vi "Preference_Panel.vi"(0 "Mode":T3) -> ()   [LabVIEW 2022 SP3]
uses:
  Anemometry Sub Vis/Controls/Server_Comms.ctl
  Anemometry Sub Vis/Controls/Preference_Mode.ctl
  Anemometry Sub Vis/Controls/GMU Gas Line Name.ctl
  Anemometry Sub Vis/File/Setup_Filetype.ctl
  Anemometry Sub Vis/Controls/Overhead.ctl
  ADAM Client/Sub VIs/ADAM Controls/Ch_description_ADAM.ctl
  ADAM Client/Sub VIs/ADAM Controls/Module_type_ADAM.ctl
  ADAM Client/Sub VIs/ADAM Controls/Function_ADAM.ctl
  ADAM Client/Sub VIs/ADAM Controls/Channel_State.ctl
  ADAM Client/Sub VIs/ADAM Controls/Calib_type_ADAM.ctl
  ADAM Client/Sub VIs/ADAM Controls/Address.ctl
  Anemometry Sub Vis/Controls/Serveds.ctl
  <vilib>/Utility/error.llb/Trim Whitespace One-Sided.vi
  Anemometry Sub Vis/Globals/Constants_global.vi
  Anemometry Sub Vis/Globals/Preference_global.vi
  <vilib>/Utility/config.llb/Read Key (Path).vi
  <vilib>/Utility/config.llb/Read Key (String).vi
  <vilib>/Utility/config.llb/Read Key (Boolean).vi
  Anemometry Sub Vis/Globals/Trav_pos_global.vi
  <vilib>/Utility/config.llb/Read Key (U32).vi
  <vilib>/Utility/config.llb/Read Key (Double).vi
  Camera Server/Globals/CamServer global.vi
  <vilib>/Utility/config.llb/Write Key (String).vi
  <vilib>/Utility/config.llb/Write Key (U32).vi
  <vilib>/Utility/config.llb/Write Key (Double).vi
  <vilib>/Utility/config.llb/Write Key (Boolean).vi
  <vilib>/Utility/config.llb/Write Key (I32).vi
  <vilib>/Utility/config.llb/Write Key (Path).vi
  <vilib>/Utility/config.llb/NI_LVConfig.lvlib
panel:
  out "siteString":string
  out "Default Gas Line Name":T1
  in  "Change?":bool
  out "User Name":string
  out "Templates folder":path
  out "Copy of Current User Preferences":path
  in  "Use New Collision Code":bool
  in  "Traverse to Traverse Collision Detection":bool
  in  "IMAQ?":bool
  in  "View Local Cameras Now":bool
  in  "Select Local Cameras to Log":i32[](listbox)
  in  "Log Cameras if available":bool
  in  "MaxDailyEmails":u32=20
  out "auditTrail":string[](array[string])
  out "currentCase":string
  out "prefsPath":path
  in  "DefaultFileExtension":string=".xls"
  in  "Post Processing Machine":bool
  in  "ADAM Setup File":u16(ring) items=["mapTest.xls", "AliGRCvac.xls", "Current_Setup.xls"]
  in  "Rig Setup":u16(ring) items=["All_Rigs", "TestRig", "--New Rig Setup--"]
  in  "Default Traverse Name":u16(ring) items=["None", "--New Traverse Setup--"]
  in  "Data Folder":path
  out "Preferences for computer":string
  in  "Reset Email Counter":bool
  in  "Default Source Establishment Time (s)":dbl=20.0
  in  "% Error From Previous Calib":dbl=0.5 format="%.1f"
  in  "Tunnel Speed Control":bool
  out "This Machine's IP Number":string
  in  "Server port number":u32=3363
  in  "Server address":string
  in  "Server Comms":T2
  in  "OK":bool
  out "Templates":path=path "/G4_2_HD/Applications (Mac OS 9)/EnFlo Software/Anemometry/Anemometry Sub Vis/Templates"
  out "EnFlo SW Preferences":path=path "/G4_2_HD/Applications (Mac OS 9)/LabVIEW 5.1/EnFlo SW Preferences"
  in  "SMTP server IP address":string
  in  "Temperature":string
  in  "Abs Press (mbar)":string
  out "LabVIEW Administrators":string[](array[string])
  in  "FixedUserName":bool caption="Auto?"
  # "Server Computer Peferences"
  # "Email Peferences"
  # "Values come from the Channel named\nLabVIEW:Administrators:\non the ADAM Scan Table. Email addesses are\n in the \"string\" box separated by semi colons."
  # "Camera Peferences"
  # "Multi Run Preferences"
  # "Warning Levels for Autocalibration Changes"
  # "Deg C"
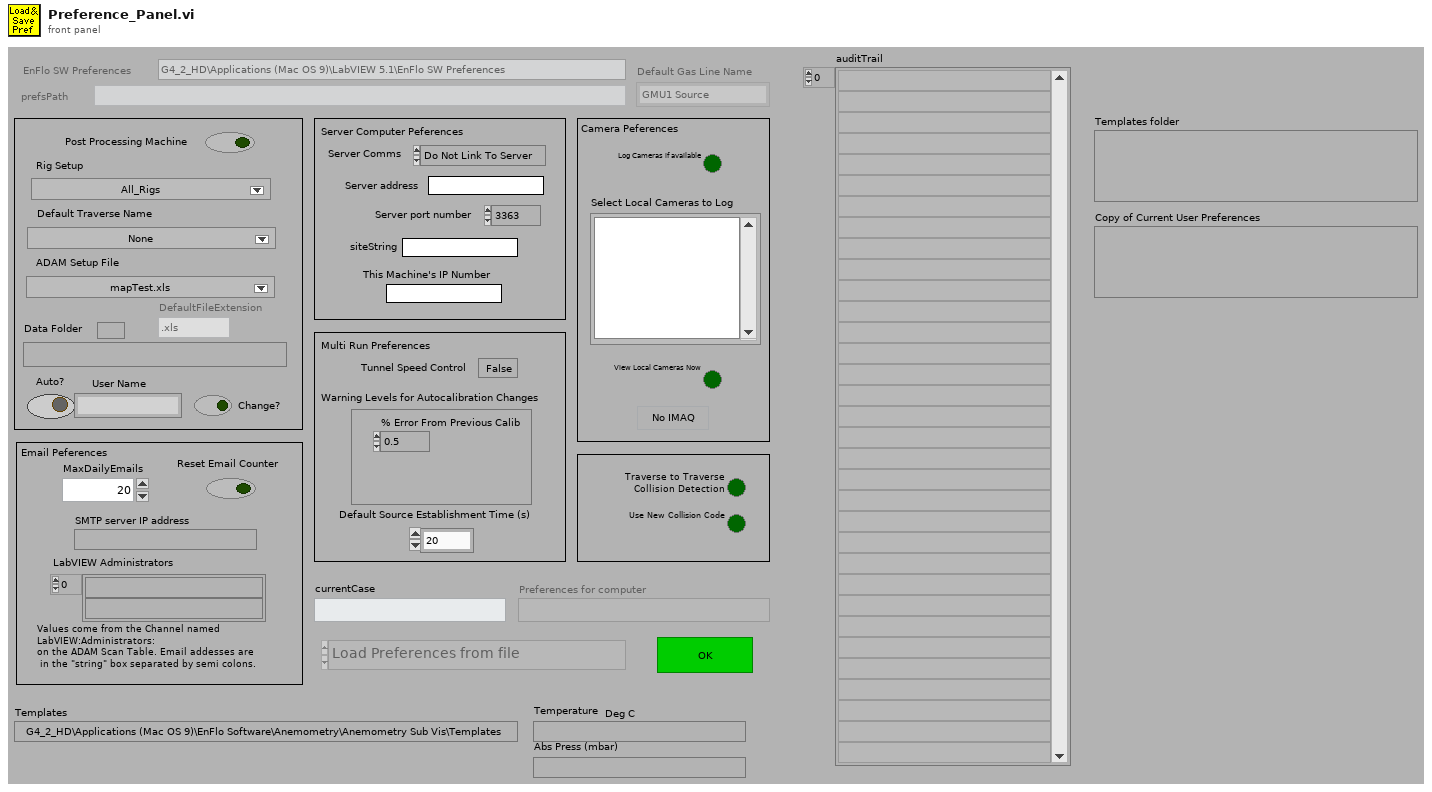
[diagram p1: front panel]
types:
  T1 = typedef "GMU Gas Line Name.ctl" = enum16{"GMU1 Source", "GMU2 Source", "GMU2 Calib", "CPP GRC-A", "CPP GRC-B"}
  T2 = typedef "Server_Comms.ctl" = enum16{"Do Not Link To Server", "Server Link Healthy"}
  T3 = typedef "Preference_Mode.ctl" = enum16{"Load Preferences from file", "Save Preferences to file", "Load, Edit then Save"}
  T4 = enum8{"Enabled", "Disabled", "Disabled and Grayed Out"}
  T5 = typedef "Setup_Filetype.ctl" = enum16{"Measurement Setups", "Calibration Setups", "General", "Results File Plotter Setups", "Speed Calib Tweaks"}
  T6 = enum16{"Zero or one", "One", "Zero or more", "One or more"}
  T7 = typedef "Overhead.ctl" = enum16{"Update total times", "Read Current Overhead", "Re Scale totals to 3 hrs", "Initialise totals to 3hr"}
  T8 = typedef "Calib_type_ADAM.ctl" = string
  T9 = typedef "Module_type_ADAM.ctl" = string
  T10 = typedef "Channel_State.ctl" = enum16{"On", "Off", "Always On", "Always Off"}
  T11 = typedef "Serveds.ctl" = enum16{"Read Global", "Load Global From File"}
  T12 = typedef "NI_LVConfig.lvlib/Config Data RefNum.ctl" = refnum<k1>
  T13 = typedef "LVDateTimeRec.ctl" = cluster{"fractional second":dbl, "second":i32, "minute":i32, "hour":i32, "day of month":i32, "month":i32, "year":i32, "day of week":i32, "day of year":i32, "DST":i32}
  T14 = typedef "camCluster.ctl" = cluster{"cam":string, "URL":string, "ADAMspecs":cluster{"channel":string, "labelText":string, "formatString":string}[]}
  T15 = typedef "Camera enum.ctl" = string
  T16 = cluster{"Label.Text":string, "date/time string":string}[]
  T17 = typedef "Ch_description_ADAM.ctl" = cluster{"Ch Name":string, "Type":T9, "Function":T18, "Ch State":T10, "Calibration type":T8, "A":dbl, "B":dbl, "C":dbl, "D":dbl, "Comments":string, "Address":T19, "String":string, "Duty":u16}
  T18 = typedef "Function_ADAM.ctl" = enum16{"Analogue Input", "Digital Input", "Event counter", "Event rate", "Analogue Output", "Digital Output", "Relay Output"}
  T19 = typedef "Address.ctl" = cluster{"Main":i32, "Ch.":i32, "Sub":i32, "Port Name":string}
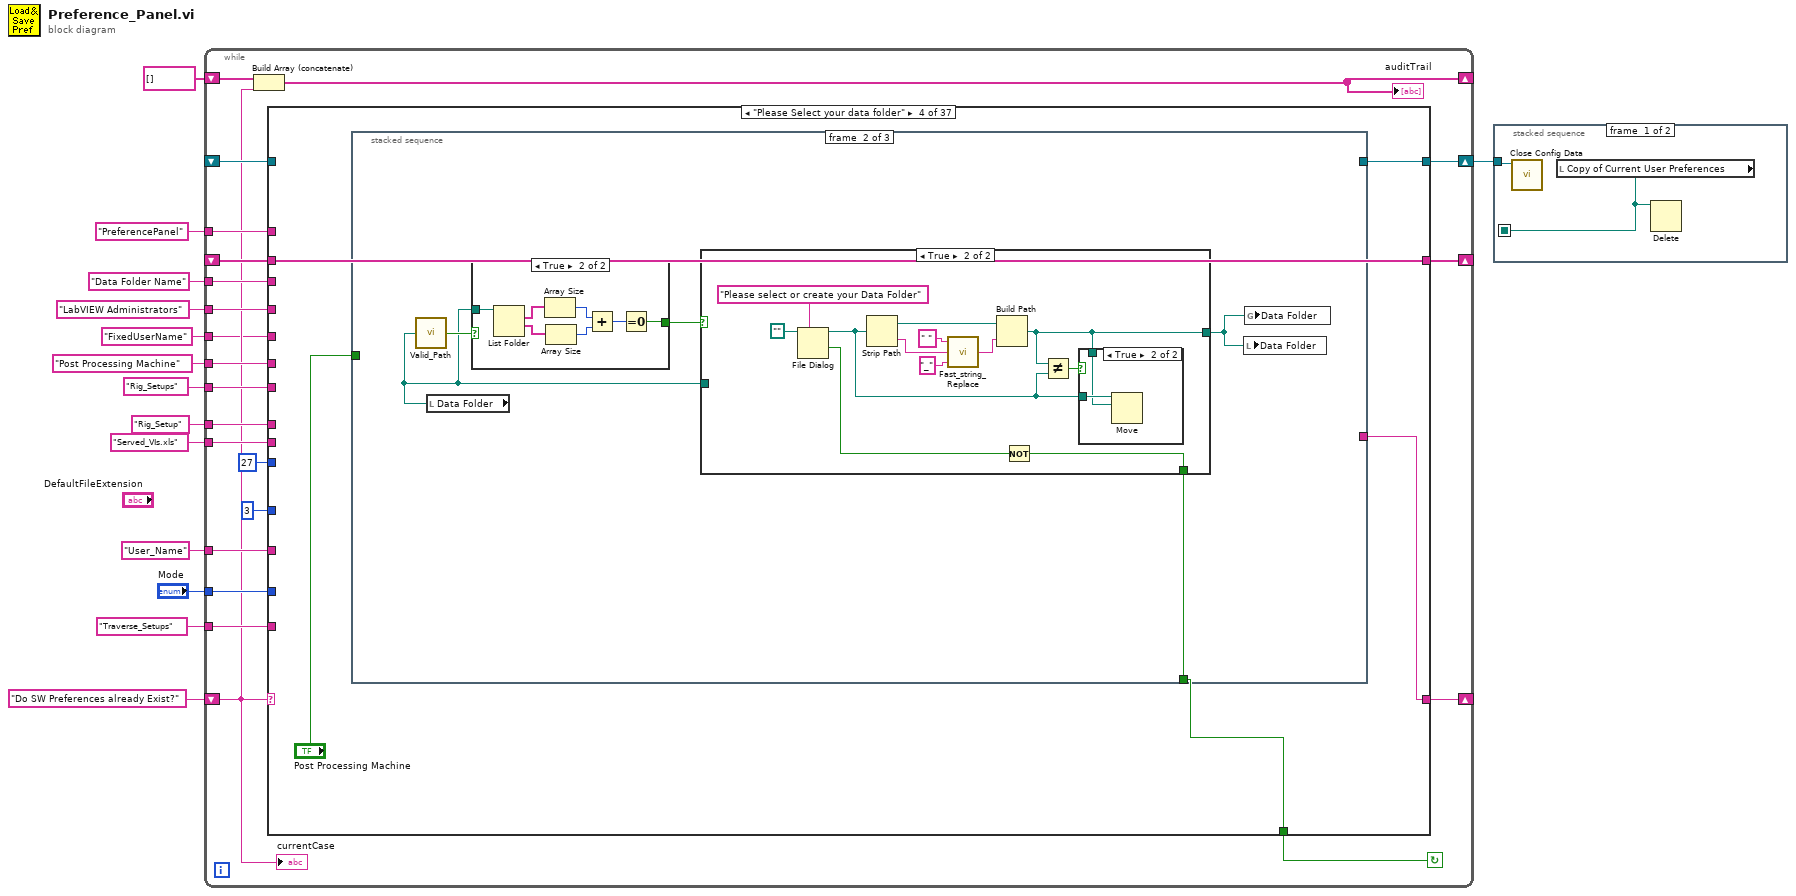
[diagram p0: block diagram]
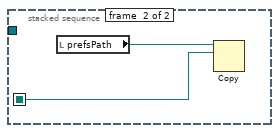
[diagram p2: hidden frame]
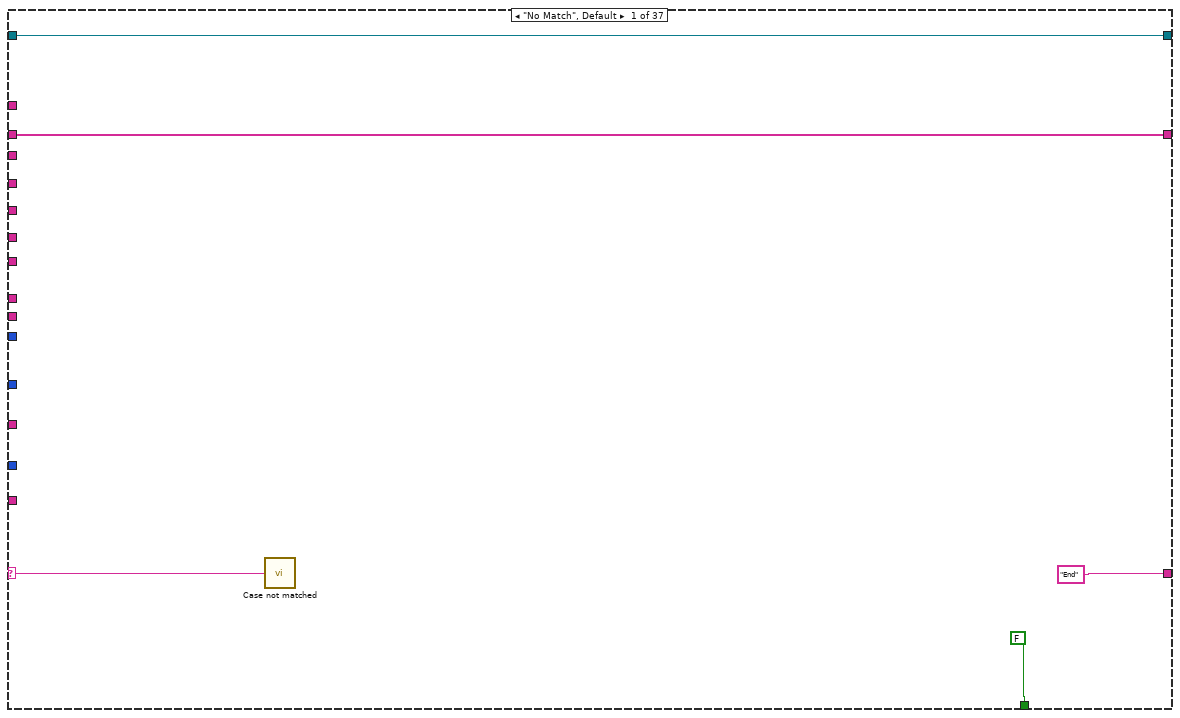
[diagram p3: hidden frame]
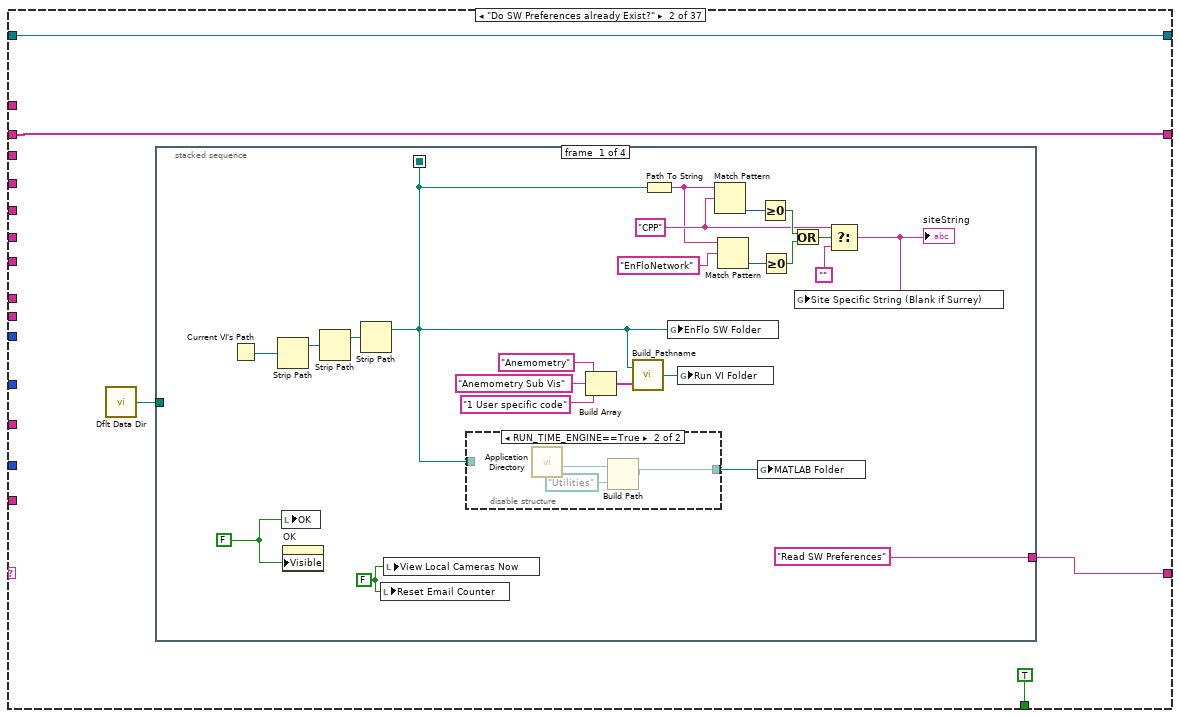
[diagram p4: hidden frame]
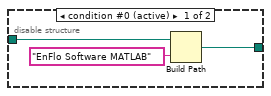
[diagram p5: hidden frame]
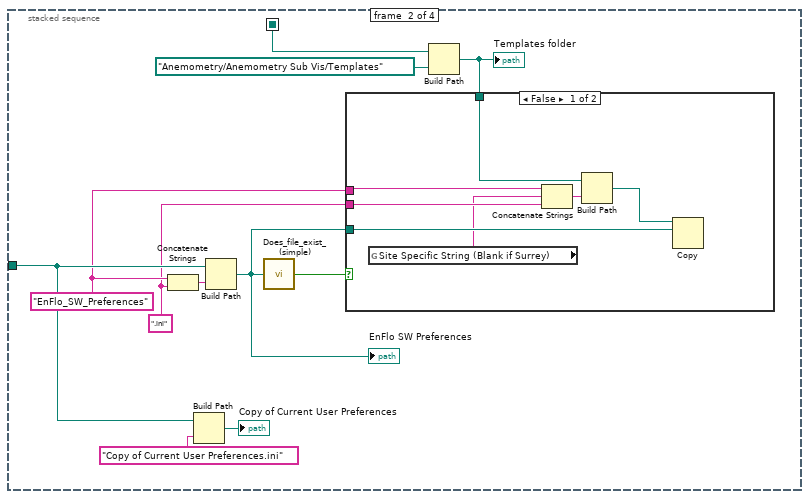
[diagram p6: hidden frame]
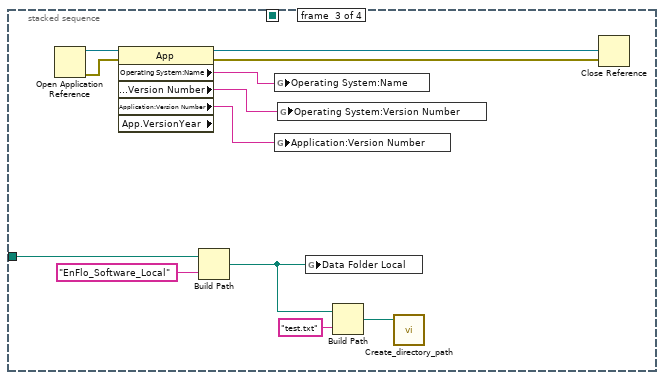
[diagram p8: hidden frame]
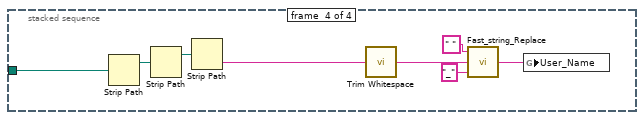
[diagram p9: hidden frame]
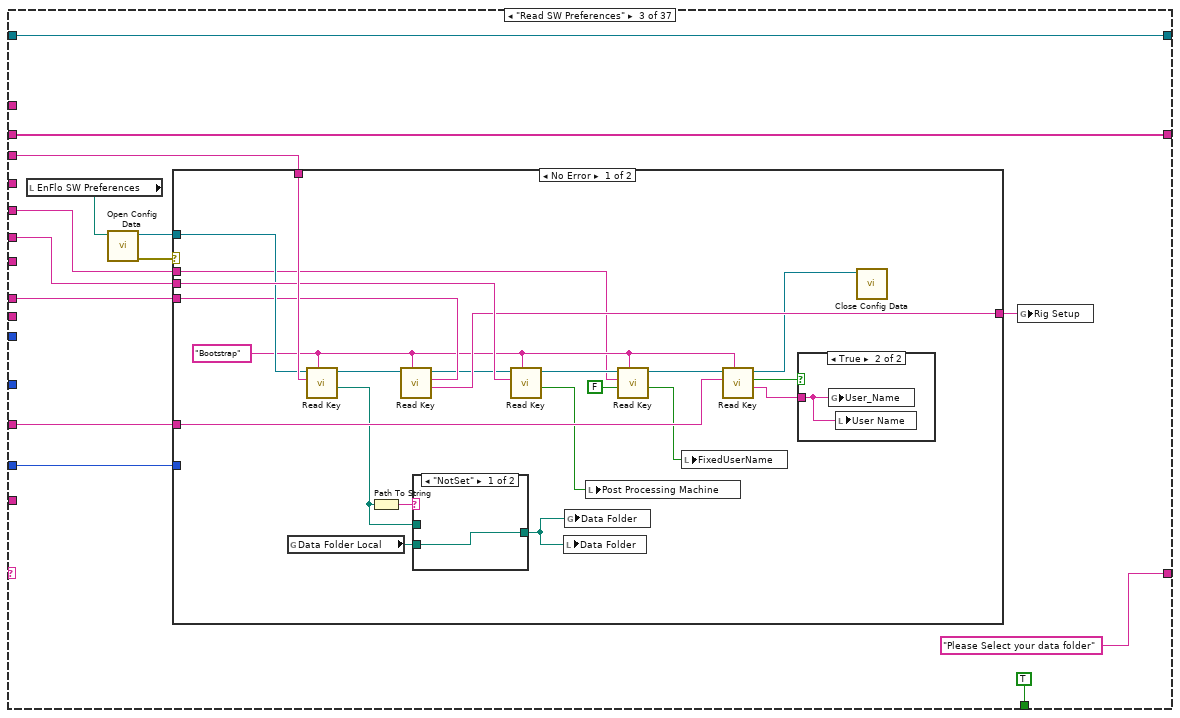
[diagram p10: hidden frame]
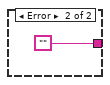
[diagram p13: hidden frame]
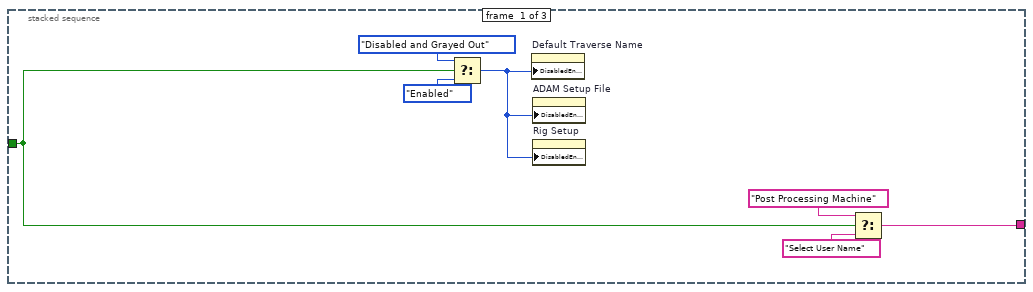
[diagram p14: hidden frame]
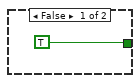
[diagram p15: hidden frame]
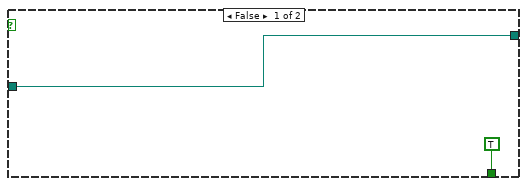
[diagram p16: hidden frame]
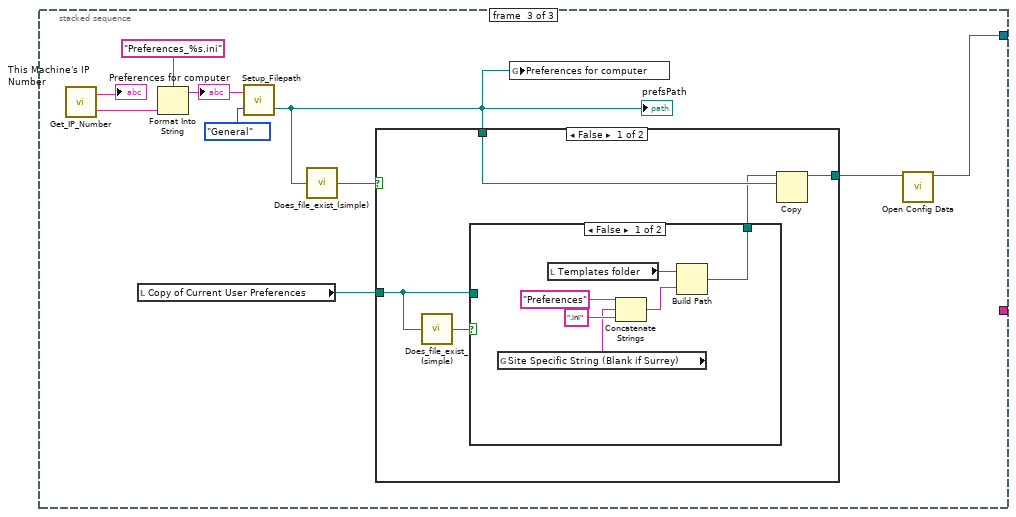
[diagram p18: hidden frame]
diagram:
  n1 = while {
    shift-left: _ -> [w34]
    shift-right: [w35] -> _
    shift-left: "Do SW Preferences already Exist?" -> [w18]
    shift-right: [w19] -> _
    tunnel: "Mode" -> [w33]
    tunnel: "Data Folder Name" ("Label for characters") -> [w32]
    tunnel: "Served_VIs.xls" ("Substring") -> [w31]
    tunnel: "Rig_Setups" ("Folder") -> [w28]
    tunnel: "Traverse_Setups" ("name or relative path") -> [w27]
    tunnel: "Post Processing Machine" ("Label for characters") -> [w26]
    tunnel: "User_Name" ("Label for characters") -> [w25]
    tunnel: "LabVIEW Administrators" -> [w24]
    tunnel: "PreferencePanel" ("section") -> [w23]
    shift-right: [w22] -> w4
    shift-left: _ -> [w21]
    tunnel: "Rig_Setup" ("Label for characters") -> [w20]
    shift-right: [w16] -> _
    shift-left: string[] [] -> [w17]
    tunnel: "FixedUserName" ("key") -> [w15]
    stop <- w36 continue-if-true
    n2 = Build Array (concatenate)(w17, w18) -> (w16:string[])
    "auditTrail" <- w16
    n3 = case shown="\"Please Select your data folder\"" w18 {
      selector: w18 -> [w37 _ _ _ _ _ _ _ _ _ _ _ _ _ _ _ _ _ _ _ _ _ _ _ _ _ _ _ _ _ _ _ _ _ _ _ _]
      tunnel: [FALSE TRUE TRUE w157 TRUE TRUE TRUE TRUE TRUE TRUE TRUE TRUE TRUE TRUE TRUE TRUE TRUE TRUE TRUE TRUE TRUE TRUE TRUE TRUE TRUE TRUE TRUE TRUE TRUE TRUE TRUE TRUE w1012 TRUE TRUE TRUE FALSE] -> w36
      tunnel: ["End" w44 "Please Select your data folder" w154 "Is rig setup blank?" w292 w298 w309 w327 "Update Constants Global" ("f") "Copy Preferences?" "Copy Preferences?" w459 w477 "Install Preference files" "Install Adam table files" "Install Adam setup files" "Choose ADAM Setup file" "Preference files continued" "Variable Names" w653 w689 "Please Enter new  Traverse Setup" w811 "Create Traverse setup" ("f") "Check file permission status" w899 w913 w933 w957 w973 "Save Preference File" "Save SW Preferences" w1134 w1148 "Initialise Globals" "End"] -> w19
      tunnel: [w39 w45 w126 w158 w227 w295 w306 w316 w329 w394 w422 w445 w458 w480 w534 w551 w577 w595 w617 w625 w658 w693 w799 w813 w848 w861 w900 w918 w938 w964 w977 w1000 w1015 w1136 w1149 w1203 w1272] -> w35
      tunnel: w34 -> [w39 w45 w126 w158 w227 w295 w306 w316 w329 w394 w422 w445 w458 w480 w534 w551 w577 w595 w617 w625 _ w693 w799 w813 w848 w861 w900 w918 w938 w964 w977 w1000 w1015 w1136 w1149 w1203 w1272]
      tunnel: w33 -> [_ _ w121 _ w222 _ _ _ _ _ _ _ _ _ _ _ _ _ _ _ w643 _ _ _ _ _ w898 _ _ _ _ _ w1013 _ _ _ _]
      tunnel: w32 -> [_ _ w125 _ w225 _ _ _ _ _ _ _ _ _ _ _ _ _ _ _ _ _ _ _ _ _ _ _ _ _ _ _ _ w1126 _ _ _]
      tunnel: w31 -> [_ _ _ _ _ _ _ _ _ _ _ _ _ _ _ w543 _ _ _ _ _ _ _ _ _ _ _ _ _ _ _ _ _ _ _ w1196 _]
      tunnel: 3 ("lower limit") -> [_ _ _ _ _ _ w303 _ w326 _ _ _ _ _ _ _ _ _ _ _ _ _ _ w810 _ _ _ _ _ _ _ _ _ _ _ _ _]
      tunnel: 27 ("upper limit") -> [_ _ _ _ _ _ w304 _ w325 _ _ _ _ _ _ _ _ _ _ _ _ _ _ w809 _ _ _ _ _ _ _ _ _ _ _ _ _]
      tunnel: w28 -> [_ _ _ _ _ _ _ _ _ w382 w411 _ _ _ _ _ _ _ _ _ _ _ _ _ _ _ _ _ _ _ _ _ _ _ _ _ _]
      tunnel: w27 -> [_ _ _ _ _ _ _ _ _ _ _ _ _ _ _ _ _ _ _ _ _ _ w797 _ w837 _ _ _ _ _ _ _ _ _ _ _ _]
      tunnel: w26 -> [_ _ w124 _ w224 _ _ _ _ _ _ _ _ _ _ _ _ _ _ _ _ _ _ _ _ _ _ _ _ _ _ _ _ w1124 _ _ _]
      tunnel: w25 -> [_ _ w122 _ w223 _ _ _ _ _ _ _ _ _ _ _ _ _ _ _ _ _ _ _ _ _ _ _ _ _ _ _ _ w1122 _ _ _]
      tunnel: w24 -> [_ _ _ _ _ _ _ _ _ _ _ _ _ _ _ _ _ _ _ _ _ _ _ _ _ _ _ _ _ _ _ _ _ _ _ _ _]
      tunnel: w23 -> [_ _ _ _ _ _ _ _ _ _ _ _ _ _ _ _ _ _ _ _ w640 w687 _ _ _ _ _ _ _ _ _ _ w1009 _ _ _ _]
      tunnel: [w38 w42 w120 w156 w221 w294 w297 w308 w321 w380 w402 w427 w450 w475 w524 w540 w562 w587 w603 w619 w638 w686 w788 w805 w834 w856 w896 w910 w930 w953 w972 w998 w1010 w1132 w1147 w1194 w1258] -> w22
      tunnel: w21 -> [w38 w42 w120 _ w221 w294 w297 w308 w321 w380 w402 w427 w450 w475 w524 w540 w562 w587 w603 w619 w638 w686 w788 w805 w834 w856 w896 w910 w930 w953 w972 w998 w1010 w1132 w1147 w1194 w1258]
      tunnel: w20 -> [_ _ w116 _ w220 _ _ _ _ _ _ _ _ _ _ _ _ _ _ _ _ _ _ _ _ _ _ _ _ _ _ _ _ w1116 _ _ _]
      tunnel: w15 -> [_ _ w114 _ _ _ _ _ _ _ _ _ _ _ _ _ _ _ _ _ _ _ _ _ _ _ _ _ _ _ _ _ _ w1112 _ _ _]
      frame "No Match", Default {
        n4 = call "Case not matched.vi"("Case Name not Matched"=w37) -> ()
      }
      frame "Do SW Preferences already Exist?" {
        n5 = call <vilib>:"Dflt Data Dir.vi"() -> ("App:Default Data Directory"=w43:path)
        n6 = stacked-sequence {
          seq-local: [w49 _ _ _] -> [_ w81 _ _]
          tunnel: ["Read SW Preferences" _ _ _] -> w44
          tunnel: w43 -> [_ w84 w97 w107]
          frame #0 {
            w51 = "CPP" ("regular expression")
            w62 = FALSE ("Reset Email Counter")
            w69 = FALSE ("OK")
            n7 = Current VI's Path() -> (path=w60:path)
            n8 = Strip Path(path=w60) -> (stripped path=w59:path)  [unwired: 1 out]
            n9 = local write "OK"(w69) -> ()
            n10 = property on="OK" class="Bool (strict)"("Visible"=w69) -> ()  [unwired: 2 in, 2 out]
            n11 = Strip Path(path=w59) -> (stripped path=w58:path)  [unwired: 1 out]
            n12 = Strip Path(path=w58) -> (stripped path=w49:path)  [unwired: 1 out]
            n13 = local write "Reset Email Counter"(w62) -> ()
            n14 = local write "View Local Cameras Now"(w62) -> ()
            n15 = disable-structure shown="RUN_TIME_ENGINE==True" {
              disable-tunnel: [w71 w75] -> w63
              disable-tunnel: w49 -> [w70 _]
              frame condition #0 (active) {
                n16 = Build Path(base path=w70, name or relative path="EnFlo Software MATLAB") -> (appended path=w71:path)
              }
              frame condition #1 {
                n17 = call <vilib>:"Application Directory.vi"() -> ("Application Directory"=w74:path)
                n18 = Build Path(base path=w74, name or relative path=path "Utilities") -> (appended path=w75:path)
              }
            }
            n19 = Build Array("Anemometry" ("name or relative path"), "Anemometry Sub Vis" ("name or relative path"), "1 User specific code" ("name or relative path")) -> (w64:string[])
            n20 = call "Build_Pathname.vi"("PathElements"=w64, "PathnameIn"=w49) -> ("AppendedPath"=w68:path)
            n21 = Path To String(path=w49) -> (string=w48:string)
            n22 = global write "Constants_global.vi" "EnFlo SW Folder"(w49) -> ()
            n23 = global write "Constants_global.vi" "Run VI Folder"(w68) -> ()
            n24 = Match Pattern(string=w48, regular expression=w51) -> (offset past match=w57:i32)  [unwired: 1 in, 3 out]
            n25 = Match Pattern(string=w48, regular expression="EnFloNetwork") -> (offset past match=w56:i32)  [unwired: 1 in, 3 out]
            n26 = global write "Constants_global.vi" "MATLAB Folder"(w63) -> ()
            n27 = Greater Or Equal To 0?(x=w57) -> (x >= 0?=w55:bool)
            n28 = Greater Or Equal To 0?(x=w56) -> (x >= 0?=w54:bool)
            n29 = Or(x=w55, y=w54) -> (x .or. y?=w53:bool)
            n30 = Select(t=w51, s=w53, f="") -> (s? t:f=w47:string)
            "siteString" <- w47
            n31 = global write "Preference_global.vi" "Site Specific String (Blank if Surrey)"(w47) -> ()
          }
          frame #1 {
            w76 = ".ini" ("name or relative path")
            w78 = "EnFlo_SW_Preferences" ("name or relative path")
            n32 = Concatenate Strings(w78, w76) -> (w77:string)
            n33 = Build Path(base path=w84, name or relative path="Copy of Current User Preferences.ini") -> (appended path=→"Copy of Current User Preferences":path)
            n34 = Build Path(base path=w84, name or relative path=w77) -> (appended path=w82:path)
            "EnFlo SW Preferences" <- w82
            n35 = call "Does_file_exist_(simple).vi"("Pathname"=w82) -> ("exists?"=w83:bool)
            n36 = Build Path(base path=w81, name or relative path=path "Anemometry/Anemometry Sub Vis/Templates" ("appended path")) -> (appended path=w79:path)
            "Templates folder" <- w79
            n37 = case shown="False" w83 {
              tunnel: w82 -> [w92 _]
              tunnel: w79 -> [w91 _]
              tunnel: w78 -> [w89 _]
              tunnel: w76 -> [w88 _]
              frame False {
                n38 = global read "Preference_global.vi" "Site Specific String (Blank if Surrey)"() -> (w87:string)
                n39 = Concatenate Strings(w89, w87, w88) -> (w90:string)
                n40 = Build Path(base path=w91, name or relative path=w90) -> (appended path=w93:path)
                n41 = Copy(10:w92, 11:w93) -> ()  [unwired: 3 in, 3 out]
              }
              frame True {
              }
            }
          }
          frame #2 {
            n42 = Open Application Reference() -> (0:w102:errorcluster, 3:w105:refnum<vi>)  [unwired: 1 in, 3 out]
            n43 = property class="App" props=["Operating System:Name", "Operating System:Version Number", "Application:Version Number", "App.VersionYear"](reference=w105, error in=w102) -> (reference out=w104:refnum<vi>, error out=w103:errorcluster, "Operating System:Name"=w99:string, "Operating System:Version Number"=w101:string, "Application:Version Number"=w100:string)  [unwired: 1 out]
            n44 = Build Path(base path=w97, name or relative path="EnFlo_Software_Local" ("element")) -> (appended path=w96:path)
            n45 = global write "Preference_global.vi" "Operating System:Name"(w99) -> ()
            n46 = global write "Preference_global.vi" "Application:Version Number"(w100) -> ()
            n47 = global write "Preference_global.vi" "Operating System:Version Number"(w101) -> ()
            n48 = global write "Constants_global.vi" "Data Folder Local"(w96) -> ()
            n49 = Build Path(base path=w96, name or relative path="test.txt") -> (appended path=w94:path)
            n50 = call "Create_directory_path.vi"("Path name"=w94) -> ()  [unwired: 2 in, 2 out]
            n51 = Close Reference(reference=w104, error in (no error)=w103) -> ()  [unwired: 1 out]
          }
          frame #3 {
            n52 = Strip Path(path=w107) -> (stripped path=w109:path)  [unwired: 1 out]
            n53 = Strip Path(path=w109) -> (stripped path=w108:path)  [unwired: 1 out]
            n54 = Strip Path(path=w108) -> (name=w106:string)  [unwired: 1 out]
            n55 = call <vilib>:"Trim Whitespace.vi"("string"=w106) -> ("trimmed string"=w110:string)  [unwired: 1 in]
            n56 = call "Fast_string_Replace.vi"("Replace match with:"="_", "Input String"=w110, "matchThis"=" " ("regular expression")) -> ("Output String"=w111:string)  [unwired: 1 in, 1 out]
            n57 = global write "Preference_global.vi" "User_Name"(w111) -> ()
          }
        }
      }
      frame "Read SW Preferences" {
        n58 = local read "EnFlo SW Preferences"() -> (w117:path)
        n59 = call <vilib>:"Open Config Data.vi"("configuration file path"=w117) -> ("error out"=w118:errorcluster, "refnum"=w119:T12)  [unwired: 8 in, 1 out]
        n60 = case shown="No Error" w118 {
          tunnel: w125 -> [w149 _]
          tunnel: w124 -> [w148 _]
          tunnel: [w147 ""] -> w123
          tunnel: w122 -> [w146 _]
          tunnel: w121 -> [_ _]
          tunnel: w119 -> [w145 _]
          tunnel: w116 -> [w144 _]
          tunnel: w114 -> [w129 _]
          frame No Error {
            w130 = "Bootstrap"
            n61 = global read "Constants_global.vi" "Data Folder Local"() -> (w136:path)
            n62 = call-poly <vilib>:"Read Key.vi"("section"=w130, "key"=w149, "refnum"=w145) -> ("value"=w134:path, "refnum out"=w140:T12)  [unwired: 5 in, 2 out]
            n63 = Path To String(path=w134) -> (string=w137:string)
            n64 = call-poly <vilib>:"Read Key.vi"("section"=w130, "key"=w144, "refnum"=w140) -> ("value"=w147:string, "refnum out"=w139:T12)  [unwired: 5 in, 2 out]
            n65 = case shown="\"NotSet\"" w137 {
              tunnel: w136 -> [w150 _]
              tunnel: [w150 w151] -> w135
              tunnel: w134 -> [_ w151]
              frame "NotSet" {
              }
              frame "Set", Default {
              }
            }
            n66 = call-poly <vilib>:"Read Key.vi"("section"=w130, "key"=w148, "refnum"=w139) -> ("value"=w143:bool, "refnum out"=w133:T12)  [unwired: 5 in, 2 out]
            n67 = local write "Data Folder"(w135) -> ()
            n68 = global write "Constants_global.vi" "Data Folder"(w135) -> ()
            n69 = local write "Post Processing Machine"(w143) -> ()
            n70 = call-poly <vilib>:"Read Key.vi"("section"=w130, "default value"=FALSE, "key"=w129, "refnum"=w133) -> ("value"=w128:bool, "refnum out"=w132:T12)  [unwired: 4 in, 2 out]
            n71 = local write "FixedUserName"(w128) -> ()
            n72 = call-poly <vilib>:"Read Key.vi"("section"=w130, "key"=w146, "refnum"=w132) -> ("value"=w141:string, "found?"=w142:bool, "refnum out"=w138:T12)  [unwired: 5 in, 1 out]
            n73 = case shown="True" w142 {
              tunnel: w141 -> [_ w152]
              frame False {
              }
              frame True {
                n74 = global write "Preference_global.vi" "User_Name"(w152) -> ()
                n75 = local write "User Name"(w152) -> ()
              }
            }
            n76 = call <vilib>:"Close Config Data.vi"("refnum"=w138) -> ()  [unwired: 9 in, 2 out]
          }
          frame Error {
          }
        }
        n77 = global write "Preference_global.vi" "Rig Setup"(w123) -> ()
      }
      frame "Please Select your data folder" {
        n78 = stacked-sequence {
          tunnel: [_ w170 _] -> w157
          tunnel: "Post Processing Machine" -> [w159 _ _]
          tunnel: [_ _ w199] -> w156
          tunnel: [w160 _ _] -> w154
          frame #0 {
            n79 = Select(t=T4."Disabled and Grayed Out" ("Disabled"), s=w159, f=T4."Enabled" ("Disabled")) -> (s? t:f=w165:T4)
            n80 = property on="Default Traverse Name" class="Ring (strict)"("DisabledEnum"=w165) -> ()  [unwired: 2 in, 2 out]
            n81 = property on="ADAM Setup File" class="Ring (strict)"("DisabledEnum"=w165) -> ()  [unwired: 2 in, 2 out]
            n82 = property on="Rig Setup" class="Ring (strict)"("DisabledEnum"=w165) -> ()  [unwired: 2 in, 2 out]
            n83 = Select(t="Post Processing Machine", s=w159, f="Select User Name") -> (s? t:f=w160:string)
          }
          frame #1 {
            n84 = local read "Data Folder"() -> (w166:path)
            n85 = call "Valid_Path.vi"("Filename"=w166) -> ("Valid Path?"=w168:bool)
            n86 = case shown="True" w168 {
              tunnel: [TRUE ("status") w172] -> w167
              tunnel: w166 -> [_ w178]
              frame False {
              }
              frame True {
                n87 = List Folder(path=w178) -> (filenames=w176:string[], folder names=w177:string[])  [unwired: 1 in, 4 out]
                n88 = Array Size(array=w176) -> (size(s)=w174:i32)
                n89 = Array Size(array=w177) -> (size(s)=w175:i32)
                n90 = Add(x=w174, y=w175) -> (x+y=w173:i32)
                n91 = Equal To 0?(x=w173) -> (x = 0?=w172:bool)
              }
            }
            n92 = case shown="True" w167 {
              tunnel: [w180 w183] -> w169
              tunnel: w166 -> [w180 _]
              tunnel: [TRUE w181] -> w170
              frame False {
              }
              frame True {
                n93 = File Dialog(7:"Please select or create your Data Folder" ("prompt"), 11:path "") -> (1:w182:bool, 3:w184:path)  [unwired: 1 in, 6 out]
                n94 = Strip Path(path=w184) -> (stripped path=w188:path, name=w187:string)
                n95 = call "Fast_string_Replace.vi"("Replace match with:"="_", "Input String"=w187, "matchThis"=" " ("regular expression")) -> ("Output String"=w186:string)  [unwired: 1 in, 1 out]
                n96 = Build Path(base path=w188, name or relative path=w186) -> (appended path=w183:path)
                n97 = Not(x=w182) -> (.not. x?=w181:bool)
                n98 = Not Equal?(x=w183, y=w184) -> (x != y?=w185:bool)
                n99 = case shown="True" w185 {
                  tunnel: w184 -> [_ w194]
                  tunnel: w183 -> [_ w193]
                  frame False {
                  }
                  frame True {
                    n100 = Move(source path=w194, 10:w193) -> ()  [unwired: 1 in, 5 out]
                  }
                }
              }
            }
            n101 = local write "Data Folder"(w169) -> ()
            n102 = global write "Constants_global.vi" "Data Folder"(w169) -> ()
          }
          frame #2 {
            n103 = call "Get_IP_Number.vi"() -> ("bestAvailableName"=w203:string, "IP Number"=→"This Machine's IP Number":string)
            n104 = local read "Copy of Current User Preferences"() -> (w196:path)
            n105 = Format Into String(format string="Preferences_%s.ini" ("name or relative path"), w203) -> (resulting string=w204:string)  [unwired: 2 in, 1 out]
            "Preferences for computer" <- w204
            n106 = call "Setup_Filepath.vi"("Setup File Type"=Setup_Filetype."General", "Filename in"=w204) -> ("Filename Out"=w195:path)  [unwired: 1 out]
            "prefsPath" <- w195
            n107 = call "Does_file_exist_(simple).vi"("Pathname"=w195) -> ("exists?"=w198:bool)
            n108 = case shown="False" w198 {
              tunnel: w195 -> [w208 w217]
              tunnel: [w209 w217] -> w197
              tunnel: w196 -> [w205 _]
              frame False {
                n109 = call "Does_file_exist_(simple).vi"("Pathname"=w205) -> ("exists?"=w207:bool)
                n110 = case shown="False" w207 {
                  tunnel: [w214 w216] -> w206
                  tunnel: w205 -> [_ w216]
                  frame False {
                    n111 = global read "Preference_global.vi" "Site Specific String (Blank if Surrey)"() -> (w210:string)
                    n112 = local read "Templates folder"() -> (w215:path)
                    n113 = Concatenate Strings("Preferences", w210, ".ini") -> (w211:string)
                    n114 = Build Path(base path=w215, name or relative path=w211) -> (appended path=w214:path)
                  }
                  frame True {
                  }
                }
                n115 = Copy(10:w208, 11:w206) -> (3:w209:path)  [unwired: 3 in, 2 out]
              }
              frame True {
              }
            }
            n116 = global write "Preference_global.vi" "Preferences for computer"(w195) -> ()
            n117 = call <vilib>:"Open Config Data.vi"("configuration file path"=w197) -> ("refnum"=w199:T12)  [unwired: 8 in, 2 out]
          }
        }
      }
      frame "Select User Name" {
        n118 = local read "Post Processing Machine"() -> (w218:bool)
        n119 = stacked-sequence {
          seq-local: [w231 _ _ _] -> [_ _ w268 _]
          seq-local: [_ w247 _ _] -> [_ _ w258 _]
          tunnel: w225 -> [_ _ _ _]
          tunnel: w224 -> [_ _ _ _]
          tunnel: w223 -> [_ _ _ _]
          tunnel: "Add New User Name" -> [w230 _ w272 _]
          tunnel: w222 -> [_ w248 _ _]
          tunnel: w220 -> [_ _ _ _]
          tunnel: w218 -> [_ w246 _ _]
          frame #0 {
            n120 = Get Date/Time In Seconds() -> (seconds since 1Jan1904=w245:timestamp)
            n121 = global read "Constants_global.vi" "Data Folder"() -> (w238:path)
            n122 = Seconds To Date/Time(time stamp (now)=w245) -> (date time rec=w244:T13)  [unwired: 1 in]
            n123 = Unbundle By Name(w244) -> ("year"=w243:i32)
            n124 = Decrement(x=w243) -> (x-1=w242:i32)
            n125 = Number To Decimal String(number=w242) -> (decimal integer string=w237:string)  [unwired: 1 in]
            n126 = Number To Decimal String(number=w243) -> (decimal integer string=w241:string)  [unwired: 1 in]
            n127 = global read "Preference_global.vi" "Rig Setup"() -> (w229:string)
            n128 = Build Path(base path=w238, name or relative path=w241) -> (appended path=w240:path)
            n129 = Build Path(base path=w238, name or relative path=w237) -> (appended path=w236:path)
            n130 = Build Path(base path=w240, name or relative path=w229) -> (appended path=w239:path)
            n131 = Build Path(base path=w236, name or relative path=w229) -> (appended path=w235:path)
            n132 = List Folder(path=w239) -> (folder names=w234:string[])  [unwired: 3 in, 3 out]
            n133 = List Folder(path=w235) -> (folder names=w233:string[])  [unwired: 3 in, 3 out]
            n134 = Build Array (concatenate)(w234, w233, w230) -> (w232:string[])
            n135 = call "Analyse_string_array.vi"("String array"=w232) -> ("Unique strings"=w231:string[])  [unwired: 1 in, 1 out]
          }
          frame #1 {
            n136 = case shown="False" w246 {
              tunnel: w248 -> [w255 _]
              tunnel: [w251 FALSE] -> w247
              frame False {
                n137 = Equal?(x=Preference_Mode."Load Preferences from file" ("Mode"), y=w255) -> (x = y?=w253:bool)
                n138 = local read "FixedUserName"() -> (w249:bool)
                n139 = Compound Arithmetic op=AND(w253, invert w249) -> (w250:bool)
                n140 = local read "Change?"() -> (w252:bool)
                n141 = Or(x=w250, y=w252) -> (x .or. y?=w251:bool)
              }
              frame True {
              }
            }
          }
          frame #2 {
            n142 = global read "Preference_global.vi" "User_Name"() -> (w269:string)
            n143 = call "Get_IP_Number.vi"() -> ("bestAvailableName"=w261:string, "IP Number"=w262:string)
            n144 = local write "This Machine's IP Number"(w262) -> ()
            n145 = Search 1D Array(1D array=w268, element=w269) -> (index of element=w267:i32)  [unwired: 1 in]
            n146 = Format Into String(format string="Preferences_%s.ini" ("name or relative path"), w261) -> (resulting string=w260:string)  [unwired: 2 in, 1 out]
            n147 = local write "Preferences for computer"(w260) -> ()
            n148 = Less Than 0?(x=w267) -> (x < 0?=w266:bool)
            n149 = Select(t=nan ("Timeout (s)"), s=w266, f=60.0 ("Timeout (s)")) -> (s? t:f=w263:dbl)
            n150 = case shown="True" w258 {
              tunnel: [w273 w280] -> w270
              tunnel: w269 -> [w273 w279]
              tunnel: w268 -> [_ w278]
              tunnel: w263 -> [_ w277]
              frame False {
              }
              frame True {
                n151 = Build Array(w279) -> (w283:string[])
                n152 = call "Select_Strings.vi"("Timeout (s)"=w277, "Available Ch names"=w278, "Message"="Please Select User Name", "Selector mode"=T6."One", "Desired Ch names (in)"=w283) -> ("Cancel"=w275:bool, "Selected Channel Names"=w281:string[], "Timed out?"=w276:bool)  [unwired: 1 out]
                n153 = Compound Arithmetic op=AND(invert w276, w275) -> (w274:bool)
                n154 = Index Array(array=w281) -> (element=w280:string)  [unwired: 1 in]
                n155 = Stop(stop? (T)=w274) -> ()
              }
            }
            n156 = Equal?(x=w270, y=w272) -> (x = y?=w271:bool)
            n157 = case shown="False" w271 {
              tunnel: [w285 w286] -> w257
              tunnel: w270 -> [w285 _]
              frame False {
              }
              frame True {
                n158 = call "Input_String_Dialog.vi"("Message to user"="Please Enter User Name") -> ("Output string"=w286:string)  [unwired: 1 in, 1 out]
              }
            }
            "User Name" <- w257
            n159 = global write "Preference_global.vi" "User_Name"(w257) -> ()
          }
          frame #3 {
            n160 = local write "Change?"(FALSE ("Change?")) -> ()
          }
        }
      }
      frame "Is rig setup blank?" {
        n161 = global read "Preference_global.vi" "Rig Setup"() -> (w289:string)
        n162 = Empty String/Path?(string/path=w289) -> (empty?=w290:bool)
        n163 = Select(t="Update Rig setup menu ring", s=w290, f="Check Rig Setup name" ("t")) -> (s? t:f=w292:string)
      }
      frame "Check Rig Setup name" {
        n164 = global read "Preference_global.vi" "Rig Setup"() -> (w299:string)
        n165 = String Length(string=w299) -> (length=w305:i32)
        n166 = In Range and Coerce(upper limit=w304, x=w305, lower limit=w303) -> (In Range?=w302:bool)  [unwired: 1 out]
        n167 = Select(t="Please Enter New Rig Name", s=w302, f="Question Data Folder") -> (s? t:f=w298:string)
      }
      frame "Question Data Folder" {
        n168 = local read "Data Folder"() -> (w315:path)
        n169 = Format Into String(format string="Is the Data Folder\n%s\nCorrect?" ("message"), w315) -> (resulting string=w313:string)  [unwired: 2 in, 1 out]
        n170 = Two Button Dialog(message=w313, 1:"No, let me change it" ("F button name (\"Cancel\")"), 2:"Yes" ("T button name (\"OK\")")) -> (T button?=w310:bool)
        n171 = case shown="True" w310 {
          tunnel: ["Please Select your data folder" "Please Enter New Rig Name"] -> w309
          frame False {
            n172 = local write "Data Folder"(path "") -> ()
          }
          frame True {
          }
        }
      }
      frame "Please Enter New Rig Name" {
        n173 = global read "Preference_global.vi" "Rig Setup"() -> (w323:string)
        n174 = String Length(string=w323) -> (length=w328:i32)
        n175 = In Range and Coerce(upper limit=w325, x=w328, lower limit=w326) -> (In Range?=w324:bool)  [unwired: 1 out]
        n176 = case shown="True" w324 {
          tunnel: w323 -> [w335 w378]
          tunnel: [w331 "Update Rig setup menu ring"] -> w327
          tunnel: [w332 w378] -> w322
          tunnel: w326 -> [w334 _]
          tunnel: w325 -> [w333 _]
          frame False {
            n177 = stacked-sequence {
              seq-local: [w336 _] -> [_ w361]
              seq-local: [w343 _] -> [_ _]
              tunnel: w335 -> [w345 _]
              tunnel: w334 -> [w356 _]
              tunnel: w333 -> [w342 w359]
              tunnel: [_ w364] -> w332
              tunnel: [w348 _] -> w331
              frame #0 {
                n178 = Match Pattern(string=w345, regular expression="-") -> (before substring=w344:string, after substring=w343:string)  [unwired: 3 out]
                n179 = String Length(string=w343) -> (length=w341:i32)
                n180 = Subtract(x=w342, y=w341) -> (x-y=w340:i32)
                n181 = Format Into String(format string="Please Enter a Rig Name.\n It must be between %d and %d Characters" ("Message to user"), w356, w340) -> (resulting string=w355:string)  [unwired: 2 in, 1 out]
                n182 = call "Input_String_Dialog.vi"("Value"=w344, "Message to user"=w355) -> ("Ok Out"=w351:bool, "Output string"=w352:string)
                n183 = call "Fast_string_Replace.vi"("Replace match with:"="_", "Input String"=w352, "matchThis"=" " ("regular expression")) -> ("Output String"=w337:string)  [unwired: 1 in, 1 out]
                n184 = Select(t="Please Enter New Rig Name", s=w351, f="Save Preference File") -> (s? t:f=w348:string)
                n185 = call "Fast_string_Replace.vi"("Replace match with:"="_", "Input String"=w337, "matchThis"="-" ("regular expression")) -> ("Output String"=w336:string)  [unwired: 1 in, 1 out]
              }
              frame #1 {
                n186 = String Length(string=w361) -> (length=w360:i32)
                n187 = Subtract(x=w359, y=w360) -> (x-y=w358:i32)
                n188 = Format Into String(format string="Please Enter a Rig Machine identifier if more than one machine per Rig.\n(Leave Blank for Rigs only using one Machine.)\nMust be less than %d Characters." ("Message to user"), w358) -> (resulting string=w357:string)  [unwired: 2 in, 1 out]
                n189 = call "Input_String_Dialog.vi"("Value"="", "Message to user"=w357) -> ("Output string"=w370:string)  [unwired: 1 out]
                n190 = call "Fast_string_Replace.vi"("Replace match with:"="_", "Input String"=w370, "matchThis"=" " ("regular expression")) -> ("Output String"=w366:string)  [unwired: 1 in, 1 out]
                n191 = call "Fast_string_Replace.vi"("Replace match with:"="_", "Input String"=w366, "matchThis"="-" ("regular expression")) -> ("Output String"=w363:string)  [unwired: 1 in, 1 out]
                n192 = Empty String/Path?(string/path=w363) -> (empty?=w365:bool)
                n193 = case shown="False" w365 {
                  tunnel: [w373 w377] -> w364
                  tunnel: w361 -> [w376 w377]
                  tunnel: w363 -> [w374 _]
                  frame False {
                    n194 = Concatenate Strings(w376, "-" ("string"), w374) -> (w373:string)
                  }
                  frame True {
                  }
                }
              }
            }
          }
          frame True {
          }
        }
        n195 = global write "Preference_global.vi" "Rig Setup"(w322) -> ()
      }
      frame "Update Rig setup menu ring" {
        n196 = local read "Data Folder"() -> (w385:path)
        n197 = Build Path(base path=w385, name or relative path="Preferences") -> (appended path=w384:path)
        n198 = Build Path(base path=w384, name or relative path=w382) -> (appended path=w383:path)
        n199 = List Folder(path=w383) -> (folder names=w381:string[])  [unwired: 1 in, 5 out]
        n200 = Build Array (concatenate)(w381, "--New Rig Setup--") -> (w387:string[])
        n201 = global read "Preference_global.vi" "Rig Setup"() -> (w391:string)
        n202 = Search 1D Array(1D array=w387, element=w391) -> (index of element=w390:i32)  [unwired: 1 out]
        n203 = case shown="-1" w390 {
          selector: w390 -> [w396 _]
          tunnel: [w396 0] -> w393
          tunnel: w387 -> [w397 w400]
          tunnel: w391 -> [_ w399]
          tunnel: [w397 w398] -> w389
          frame 0, Default {
          }
          frame -1 {
            n204 = Build Array (concatenate)(w399, w400) -> (w398:string[])
          }
        }
        n205 = local write "Rig Setup"(w393) -> ()
        n206 = property on="Rig Setup" class="Ring (strict)"("Strings []"=w389) -> ()  [unwired: 2 in, 2 out]
      }
      frame "Update Constants Global" {
        n207 = global read "Constants_global.vi" "Data Folder"() -> (w409:path)
        n208 = Build Path(base path=w409, name or relative path="Preferences") -> (appended path=w412:path)
        n209 = global read "Preference_global.vi" "Rig Setup"() -> (w410:string)
        n210 = Build Path(base path=w412, name or relative path=w411) -> (appended path=w413:path)
        n211 = Build Path(base path=w413, name or relative path=w410) -> (appended path=w407:path)
        n212 = Build Path(base path=w407, name or relative path="ADAM table") -> (appended path=w417:path)
        n213 = Build Path(base path=w407, name or relative path="Serial") -> (appended path=w416:path)
        n214 = Build Path(base path=w407, name or relative path="All_Users") -> (appended path=w406:path)
        n215 = Build Path(base path=w412, name or relative path="Traverse_Setups") -> (appended path=w403:path)
        n216 = Build Path(base path=w406, name or relative path="Collision_detection") -> (appended path=w404:path)
        n217 = global write "Constants_global.vi" "ADAM setups folder"(w417) -> ()
        n218 = global write "Constants_global.vi" "Collision_detection"(w404) -> ()
        n219 = global write "Constants_global.vi" "Serial setups folder"(w416) -> ()
        n220 = global write "Constants_global.vi" "All_Users"(w406) -> ()
        n221 = global write "Constants_global.vi" "Traverse folder"(w403) -> ()
        n222 = Build Array(w403, w417, w416, w406) -> (w415:path[])
        n223 = for {
          tunnel: w415 -> [w426] mode=indexing
          n224 = Build Path(base path=w426, name or relative path="Test") -> (appended path=w424:path)
          n225 = call "Create_directory_path.vi"("Path name"=w424) -> ()  [unwired: 2 in, 2 out]
        }
      }
      frame "Post Processing Machine" {
        n226 = global read "Constants_global.vi" "Data Folder Local"() -> (w435:path)
        n227 = global read "Preference_global.vi" "User_Name"() -> (w430:string)
        n228 = Build Path(base path=w435, name or relative path="Preferences") -> (appended path=w436:path)
        n229 = Build Path(base path=w436, name or relative path=w430) -> (appended path=w431:path)
        n230 = Build Path(base path=w436, name or relative path="Traverse_Setups") -> (appended path=w428:path)
        n231 = Build Path(base path=w431, name or relative path="ADAM table") -> (appended path=w440:path)
        n232 = Build Path(base path=w431, name or relative path="Serial") -> (appended path=w439:path)
        n233 = Build Path(base path=w431, name or relative path="All_Users") -> (appended path=w432:path)
        n234 = global write "Constants_global.vi" "ADAM setups folder"(w440) -> ()
        n235 = global write "Constants_global.vi" "Serial setups folder"(w439) -> ()
        n236 = global write "Constants_global.vi" "Traverse folder"(w428) -> ()
        n237 = local write "Post Processing Machine"(TRUE ("Post Processing Machine")) -> ()
        n238 = global write "Constants_global.vi" "All_Users"(w432) -> ()
        n239 = global write "Preference_global.vi" "Rig Setup"("Post_Processing_Machine" ("Rig Setup")) -> ()
        n240 = Build Array(w428, w440, w439, w432) -> (w438:path[])
        n241 = for {
          tunnel: w438 -> [w449] mode=indexing
          n242 = Build Path(base path=w449, name or relative path="Test") -> (appended path=w447:path)
          n243 = call "Create_directory_path.vi"("Path name"=w447) -> ()  [unwired: 2 in, 2 out]
        }
      }
      frame "Copy Preferences?" {
        n244 = local read "Preferences for computer"() -> (w452:string)
        n245 = call "Setup_Filepath.vi"("Setup File Type"=Setup_Filetype."General", "Filename in"=w452) -> ("Filename Out"=w455:path)  [unwired: 1 out]
        n246 = call <vilib>:"Check if File or Folder Exists.vi"("path"=w455) -> ("file or folder exists?"=w454:bool)  [unwired: 1 in, 9 out]
        n247 = case shown="True" w454 {
          tunnel: w455 -> [w465 _]
          tunnel: [w463 TRUE ("file or folder exists?")] -> w453
          frame False {
            n248 = Strip Path(path=w465) -> (stripped path=w468:path)  [unwired: 1 out]
            n249 = Build Path(base path=w468, name or relative path="Preferences.ini") -> (appended path=w467:path)
            n250 = Move(source path=w467, 10:w465) -> (3:w464:path)  [unwired: 3 in, 2 out]
            n251 = call <vilib>:"Check if File or Folder Exists.vi"("path"=w464) -> ("file or folder exists?"=w463:bool)  [unwired: 1 in, 9 out]
          }
          frame True {
          }
        }
        n252 = global read "Preference_global.vi" "LabVIEW Administrators"() -> (→"LabVIEW Administrators":string[])
        n253 = case shown="True" w453 {
          tunnel: [w470 TRUE ("Error?")] -> w457
          frame False {
            n254 = global read "Constants_global.vi" "All_Users"() -> (w472:path)
            n255 = Build Path(base path=w472, name or relative path="Current_Username") -> (appended path=w473:path)
            n256 = call "Read_File_Simple.vi"("Filename"=w473) -> ("Error?"=w470:bool)  [unwired: 4 in, 5 out]
          }
          frame True {
          }
        }
        n257 = Select(t="Install Generic Meas Setup file", s=w457, f="Copy from last user") -> (s? t:f=w459:string)
      }
      frame "Copy from last user" {
        n258 = stacked-sequence {
          seq-local: [w482 _ _ _] -> [_ w499 w508 w520]
          seq-local: [_ w495 _ _] -> [_ _ _ w514]
          seq-local: [_ _ w503 _] -> [_ _ _ w513]
          tunnel: [_ _ _ w512] -> w479
          frame #0 {
            n259 = global read "Constants_global.vi" "All_Users"() -> (w493:path)
            n260 = Seconds To Date/Time() -> (date time rec=w489:T13)  [unwired: 2 out]
            n261 = Unbundle By Name(w489) -> ("year"=w490:i32)
            n262 = Build Path(base path=w493, name or relative path="Current_Username") -> (appended path=w491:path)
            n263 = global read "Constants_global.vi" "Data Folder"() -> (w488:path)
            n264 = global read "Preference_global.vi" "Rig Setup"() -> (w485:string)
            n265 = Number To Decimal String(number=w490) -> (decimal integer string=w487:string)  [unwired: 1 out]
            n266 = call "Read_File_Simple.vi"("Filename"=w491) -> ("string"=w484:string)  [unwired: 4 in, 5 out]
            n267 = Build Array(w487, w485, w484, "Preferences" ("name or relative path")) -> (w486:string[])
            n268 = call "Build_Pathname.vi"("PathElements"=w486, "PathnameIn"=w488) -> ("AppendedPath"=w482:path)
          }
          frame #1 {
            n269 = local read "Preferences for computer"() -> (w494:string)
            n270 = Build Path(base path=w499, name or relative path="General") -> (appended path=w501:path)
            n271 = Build Path(base path=w501, name or relative path=w494) -> (appended path=w500:path)
            n272 = call "Setup_Filepath.vi"("Setup File Type"=Setup_Filetype."General", "Filename in"=w494) -> ("Filename Out"=w497:path)  [unwired: 1 out]
            n273 = Copy(10:w497, 11:w500) -> (0:w496:errorcluster)  [unwired: 3 in, 2 out]
            n274 = Unbundle By Name(w496) -> ("status"=w495:bool)
          }
          frame #2 {
            w506 = "Current_Setup.xls"
            n275 = Build Path(base path=w508, name or relative path="Meas Setups") -> (appended path=w510:path)
            n276 = Build Path(base path=w510, name or relative path=w506) -> (appended path=w509:path)
            n277 = call "Setup_Filepath.vi"("Setup File Type"=Setup_Filetype."Measurement Setups", "Filename in"=w506) -> ("Filename Out"=w505:path)  [unwired: 1 out]
            n278 = Copy(10:w505, 11:w509) -> (0:w504:errorcluster)  [unwired: 3 in, 2 out]
            n279 = Unbundle By Name(w504) -> ("status"=w503:bool)
          }
          frame #3 {
            w518 = "Current_Setup.xls"
            n280 = Build Path(base path=w520, name or relative path="Calib Setups") -> (appended path=w522:path)
            n281 = Build Path(base path=w522, name or relative path=w518) -> (appended path=w521:path)
            n282 = call "Setup_Filepath.vi"("Setup File Type"=Setup_Filetype."Calibration Setups", "Filename in"=w518) -> ("Filename Out"=w517:path)  [unwired: 1 out]
            n283 = Copy(10:w517, 11:w521) -> (0:w516:errorcluster)  [unwired: 3 in, 2 out]
            n284 = Unbundle By Name(w516) -> ("status"=w515:bool)
            n285 = Compound Arithmetic op=OR(w515, w514, w513) -> (w512:bool)
          }
        }
        n286 = Select(t="Install Generic Meas Setup file", s=w479, f="Read SW Preferences") -> (s? t:f=w477:string)
      }
      frame "Install Generic Meas Setup file" {
        n287 = global read "Constants_global.vi" "Run VI Folder"() -> (w533:path)
        n288 = Strip Path(path=w533) -> (stripped path=w531:path)  [unwired: 1 out]
        n289 = Build Path(base path=w531, name or relative path="Templates") -> (appended path=w529:path)
        "Templates" <- w529
        n290 = call "Setup_Filepath.vi"("Setup File Type"=Setup_Filetype."Measurement Setups", "Filename in"="Current_Setup.xls" ("name or relative path")) -> ("Filename Out"=w525:path)  [unwired: 1 out]
        n291 = call "Does_file_exist_(simple).vi"("Pathname"=w525) -> ("exists?"=w530:bool)
        n292 = case shown="False" w530 {
          tunnel: w525 -> [w539 _]
          tunnel: w529 -> [w537 _]
          frame False {
            n293 = Build Path(base path=w537, name or relative path="Measurement Setup.xls") -> (appended path=w536:path)
            n294 = Copy(10:w539, 11:w536) -> ()  [unwired: 1 in, 5 out]
          }
          frame True {
          }
        }
      }
      frame "Install Preference files" {
        n295 = local read "Preferences for computer"() -> (w546:string)
        n296 = Build Array("Preferences.xls", w543, "Month_Names.xls" ("name or relative path"), "LDA_Configuration.xls") -> (w541:string[])
        n297 = Build Array(w546, w543, "Month_Names.xls" ("name or relative path"), "LDA_Configuration.xls") -> (w550:string[])
        n298 = for {
          tunnel: w550 -> [w555] mode=indexing
          tunnel: w541 -> [w553] mode=indexing
          n299 = call "Setup_Filepath.vi"("Setup File Type"=Setup_Filetype."General", "Filename in"=w555) -> ("Filename Out"=w554:path)  [unwired: 1 out]
          n300 = call "Does_file_exist_(simple).vi"("Pathname"=w554) -> ("exists?"=w557:bool)
          n301 = case shown="False" w557 {
            tunnel: w554 -> [w561 _]
            tunnel: w553 -> [w558 _]
            frame False {
              n302 = local read "Templates"() -> (w559:path)
              n303 = Build Path(base path=w559, name or relative path=w558) -> (appended path=w560:path)
              n304 = Copy(10:w561, 11:w560) -> ()  [unwired: 1 in, 5 out]
            }
            frame True {
            }
          }
        }
      }
      frame "Install Adam table files" {
        w567 = "Current_Setup.xls"
        n305 = global read "Constants_global.vi" "ADAM setups folder"() -> (w569:path)
        n306 = Build Path(base path=w569, name or relative path="Setup_Files") -> (appended path=w565:path)
        n307 = Build Path(base path=w565, name or relative path=w567) -> (appended path=w564:path)
        n308 = Build Path(base path=w569, name or relative path=w567) -> (appended path=w570:path)
        n309 = call "Create_directory_path.vi"("Path name"=w564) -> ("Path name Out"=w563:path)  [unwired: 2 in, 1 out]
        n310 = Move(source path=w570, 10:w563) -> ()  [unwired: 1 in, 5 out]
        n311 = Build Array("Hi_Tec_Calibs.xls" ("name or relative path"), "A_Tunnel DB setup.xls" ("Substring"), "EnFlo_Tunnel DB setup.xls", "Aero_Tunnel DB setup.xls" ("name or relative path"), "D_Tunnel DB setup.xls") -> (w576:string[])
        n312 = for {
          tunnel: w576 -> [w580] mode=indexing
          tunnel: w569 -> [w581]
          n313 = Build Path(base path=w581, name or relative path=w580) -> (appended path=w579:path)
          n314 = call "Does_file_exist_(simple).vi"("Pathname"=w579) -> ("exists?"=w582:bool)
          n315 = case shown="False" w582 {
            tunnel: w579 -> [w586 _]
            tunnel: w580 -> [w583 _]
            frame False {
              n316 = local read "Templates"() -> (w584:path)
              n317 = Build Path(base path=w584, name or relative path=w583) -> (appended path=w585:path)
              n318 = Copy(10:w586, 11:w585) -> ()  [unwired: 1 in, 5 out]
            }
            frame True {
            }
          }
        }
      }
      frame "Install Adam setup files" {
        w591 = "Current_Setup.xls"
        n319 = global read "Constants_global.vi" "ADAM setups folder"() -> (w593:path)
        n320 = Build Path(base path=w593, name or relative path="Setup_Files") -> (appended path=w590:path)
        n321 = Build Path(base path=w590, name or relative path=w591) -> (appended path=w588:path)
        n322 = call "Does_file_exist_(simple).vi"("Pathname"=w588) -> ("exists?"=w589:bool)
        n323 = case shown="False" w589 {
          tunnel: w588 -> [w602 _]
          tunnel: w591 -> [w600 _]
          frame False {
            n324 = local read "Templates"() -> (w601:path)
            n325 = Build Path(base path=w601, name or relative path="ADAM_Setup_files") -> (appended path=w599:path)
            n326 = Build Path(base path=w599, name or relative path=w600) -> (appended path=w598:path)
            n327 = Copy(10:w602, 11:w598) -> ()  [unwired: 1 in, 5 out]
          }
          frame True {
          }
        }
      }
      frame "Choose ADAM Setup file" {
        w611 = "Selected_Filename.txt" ("Substring")
        n328 = global read "Constants_global.vi" "ADAM setups folder"() -> (w615:path)
        n329 = Build Path(base path=w615, name or relative path="Setup_Files") -> (appended path=w612:path)
        n330 = Build Array(w611) -> (w613:string[])
        n331 = Build Path(base path=w612, name or relative path=w611) -> (appended path=w610:path)
        n332 = call "List_files_in_order_of_age.vi"("Files to Hide"=w613, "Folder"=w612) -> ("file names"=w609:string[])  [unwired: 9 in]
        n333 = call "Read_File_Simple.vi"("Filename"=w610) -> ("string"=w608:string)  [unwired: 2 in, 7 out]
        n334 = Search 1D Array(1D array=w609, element=w608) -> (index of element=w605:i32)  [unwired: 1 out]
        n335 = property on="ADAM Setup File" class="Ring (strict)"("Strings []"=w609) -> ()  [unwired: 2 in, 2 out]
        n336 = Less Than 0?(x=w605) -> (x < 0?=w606:bool)
        n337 = Select(t=0, s=w606, f=w605) -> (s? t:f=w604:i32)
        n338 = local write "ADAM Setup File"(w604) -> ()
      }
      frame "Preference files continued" {
        n339 = Build Array("Hot_Wire_Bridges.txt", "Hot_Wire_Probes.txt", "Pressure_Transducers.txt") -> (w620:string[])
        n340 = for {
          tunnel: w620 -> [w628] mode=indexing
          n341 = call "Setup_Filepath.vi"("Setup File Type"=Setup_Filetype."Calibration Setups", "Filename in"=w628) -> ("Filename Out"=w627:path)  [unwired: 1 out]
          n342 = call "Does_file_exist_(simple).vi"("Pathname"=w627) -> ("exists?"=w630:bool)
          n343 = case shown="False" w630 {
            tunnel: w627 -> [w634 _]
            tunnel: w628 -> [w631 _]
            frame False {
              n344 = local read "Templates"() -> (w632:path)
              n345 = Build Path(base path=w632, name or relative path=w631) -> (appended path=w633:path)
              n346 = Copy(10:w634, 11:w633) -> ()  [unwired: 1 in, 5 out]
            }
            frame True {
            }
          }
        }
      }
      frame "Variable Names" {
        w639 = "HaveIMAQlib" ("key")
        n347 = local read "Post Processing Machine"() -> (w641:bool)
        n348 = local read "siteString"() -> (w635:string)
        n349 = call-poly <vilib>:"Read Key.vi"("section"=w640, "key"=w639, "refnum"=w638) -> ("value"=w636:bool)  [unwired: 5 in, 3 out]
        n350 = case shown="False" w641 {
          tunnel: w636 -> [w663 _]
          tunnel: w635 -> [w662 _]
          frame False {
            # "Not PPing- might want cameras"
            n351 = case shown="False" w663 {
              tunnel: w662 -> [w664 _]
              frame False {
                # "Not using IMAQlib"
                n352 = case shown="\"CPP\"" w664 {
                  frame "False", Default {
                  }
                  frame "CPP" {
                    # "In case someone else wants to do it different..."
                    n353 = global read "Constants_global.vi" "All_Users"() -> (w670:path)
                    n354 = Build Path(base path=w670, name or relative path="WebcamsNew.ini") -> (appended path=w668:path)
                    n355 = call "getCamPrefs.vi"("INIfilePath"=w668) -> ("Array"=w667:T14[])  [unwired: 9 in, 1 out]
                    n356 = for {
                      tunnel: w667 -> [w673] mode=indexing
                      tunnel: [w672] -> w666 mode=indexing
                      tunnel: [w671] -> w665 mode=indexing
                      i -> [w671]
                      n357 = Unbundle By Name(w673) -> ("cam"=w672:string)
                    }
                    n358 = property on="Select Local Cameras to Log" class="LstBox (strict)"("Item Names"=w666, "Value"=w665) -> ()  [unwired: 2 in, 2 out]
                  }
                }
              }
              frame True {
                # "Get names of available IMAQ cameras"
                n359 = while {
                  shift-right: [w676] -> _
                  shift-left: _ -> [w675]
                  stop <- TRUE stop-if-true
                  n360 = case shown="No Error" w675 {
                    selector: w675 -> [_ w679]
                    tunnel: [w677 w679] -> w676
                    frame No Error {
                      n361 = call "Get_Available_Cameras.vi"() -> ("error out"=w677:errorcluster, "Cameras"=w678:string[])  [unwired: 2 in]
                      n362 = property on="Select Local Cameras to Log" class="LstBox (strict)"("Item Names"=w678) -> ()  [unwired: 2 in, 2 out]
                    }
                    frame Error {
                    }
                  }
                }
              }
            }
          }
          frame True {
            # "Dont try to find cameras if postprocessing"
          }
        }
        n363 = case shown="\"Load Preferences from file\"" w643 {
          tunnel: ["Load From Preference file" w681 "Save Preference File"] -> w653
          frame "Load Preferences from file" {
          }
          frame "Load, Edit then Save" {
            n364 = local read "OK"() -> (w684:bool)
            n365 = Select(t="Save Preference File", s=w684, f="Load From Preference file") -> (s? t:f=w681:string)
          }
          frame "Save Preferences to file" {
          }
        }
        n366 = Build Array("Traverse to Traverse Collision Detection", "Server address", "Server port number", "SMTP server IP address", "Server Comms", "Default Source Establishment Time (s)", "Temperature", "Abs Press (mbar)", "Default Traverse Name", "Tunnel Speed Control", "Current Overhead Factor", "EnFlo_Data_Central_Repository", "Auto Calib Error fr Previous", "Use Triangle and Tree Collision Code", "Log Cameras if available", "Local Cameras to Log", w639, "MaxEmailsPerDay") -> (w658:string[])
      }
      frame "Load From Preference file" {
        n367 = for {
          tunnel: w693 -> [w696] mode=indexing
          tunnel: w686 -> [w695]
          tunnel: w687 -> [w694]
          n368 = case shown="\"Local Cameras to Log\"" w696 {
            selector: w696 -> [w697 w700 w704 w708 w713 w717 w721 w725 w729 w733 w744 w756 w760 w764 w768 w772 w777 w781 w786]
            tunnel: w695 -> [_ w701 w706 w710 w714 w718 w722 w726 w730 w734 w745 w757 w761 w765 w769 w773 w778 w782 w787]
            tunnel: w694 -> [_ w699 w703 w707 w711 w715 w719 w723 w727 w731 w742 w755 w758 w762 w766 w770 w775 w780 w785]
            frame "No Match", Default {
              n369 = call "Was_string_matched.vi"("Match Error"=TRUE, "Variable name"=w697) -> ()  [unwired: 1 in]
            }
            frame "Server address" {
              n370 = call-poly <vilib>:"Read Key.vi"("section"=w699, "key"=w700, "refnum"=w701) -> ("value"=w702:string)  [unwired: 5 in, 3 out]
              n371 = global write "Preference_global.vi" "Server address"(w702) -> ()
              n372 = local write "Server address"(w702) -> ()
            }
            frame "Default Traverse Name" {
              n373 = call-poly <vilib>:"Read Key.vi"("section"=w703, "key"=w704, "refnum"=w706) -> ("value"=w705:string)  [unwired: 5 in, 3 out]
              n374 = global write "Trav_pos_global.vi" "Default Traverse Setup"(w705) -> ()
            }
            frame "Server port number" {
              n375 = call-poly <vilib>:"Read Key.vi"("section"=w707, "key"=w708, "refnum"=w710) -> ("value"=w709:u32)  [unwired: 5 in, 3 out]
              n376 = local write "Server port number"(w709) -> ()
              n377 = global write "Preference_global.vi" "Server port number"(w709) -> ()
            }
            frame "Default Source Establishment Time (s)" {
              n378 = call-poly <vilib>:"Read Key.vi"("section"=w711, "key"=w713, "refnum"=w714) -> ("value"=w712:dbl)  [unwired: 5 in, 3 out]
              n379 = global write "Preference_global.vi" "Default Source Establishment Time (s)"(w712) -> ()
              n380 = local write "Default Source Establishment Time (s)"(w712) -> ()
            }
            frame "Tunnel Speed Control" {
              n381 = call-poly <vilib>:"Read Key.vi"("section"=w715, "key"=w717, "refnum"=w718) -> ("value"=w716:bool)  [unwired: 5 in, 3 out]
              n382 = local write "Tunnel Speed Control"(w716) -> ()
              n383 = global write "Preference_global.vi" "Tunnel Speed Control"(w716) -> ()
            }
            frame "Traverse to Traverse Collision Detection" {
              n384 = call-poly <vilib>:"Read Key.vi"("section"=w719, "key"=w721, "refnum"=w722) -> ("value"=w720:bool)  [unwired: 5 in, 3 out]
              n385 = global write "Preference_global.vi" "Traverse to Traverse Collision Detection"(w720) -> ()
              n386 = local write "Traverse to Traverse Collision Detection"(w720) -> ()
            }
            frame "Log Cameras if available" {
              n387 = call-poly <vilib>:"Read Key.vi"("section"=w723, "key"=w725, "refnum"=w726) -> ("value"=w724:bool)  [unwired: 5 in, 3 out]
              n388 = local write "Log Cameras if available"(w724) -> ()
              n389 = global write "Preference_global.vi" "Log Cameras if available"(w724) -> ()
            }
            frame "Use Triangle and Tree Collision Code" {
              n390 = call-poly <vilib>:"Read Key.vi"("section"=w727, "key"=w729, "refnum"=w730) -> ("value"=w728:bool)  [unwired: 5 in, 3 out]
              n391 = local write "Use New Collision Code"(w728) -> ()
              n392 = global write "Preference_global.vi" "Use New Collision Code"(w728) -> ()
            }
            frame "Local Cameras to Log" {
              n393 = call-poly <vilib>:"Read Key.vi"("section"=w731, "key"=w733, "refnum"=w734) -> ("value"=w732:string)  [unwired: 5 in, 3 out]
              n394 = property on="Select Local Cameras to Log" class="LstBox (strict)"() -> ("Item Names"=w735:string[])  [unwired: 2 in, 2 out]
              n395 = call "Get_array_values_fr_String.vi"("String Value"=w732) -> ("String array"=w737:string[])  [unwired: 1 out]
              n396 = for {
                tunnel: w737 -> [w741] mode=indexing
                tunnel: w735 -> [w740]
                tunnel: [w739] -> w736 mode=indexing if=w738
                n397 = Search 1D Array(1D array=w740, element=w741) -> (index of element=w739:i32)  [unwired: 1 in]
                n398 = Greater Or Equal To 0?(x=w739) -> (x >= 0?=w738:bool)
              }
              n399 = local write "Select Local Cameras to Log"(w736) -> ()
              n400 = global write "CamServer global.vi" "Demanded Local cameras"(w737) -> ()
            }
            frame "SMTP server IP address" {
              n401 = call-poly <vilib>:"Read Key.vi"("section"=w742, "key"=w744, "refnum"=w745) -> ("value"=w743:string)  [unwired: 5 in, 3 out]
              n402 = local write "SMTP server IP address"(w743) -> ()
              n403 = global write "Preference_global.vi" "SMTP server IP address"(w743) -> ()
            }
            frame "Server Comms" {
              w750 = 6 ("length (rest)")
              n404 = local read "This Machine's IP Number"() -> (w751:string)
              n405 = call-poly <vilib>:"Read Key.vi"("section"=w755, "key"=w756, "refnum"=w757) -> ("value"=w748:u32)  [unwired: 5 in, 3 out]
              n406 = local read "Server address"() -> (w752:string)
              n407 = String Subset(string=w751, length (rest)=w750) -> (substring=w754:string)  [unwired: 1 in]
              n408 = String Subset(string=w752, length (rest)=w750) -> (substring=w753:string)  [unwired: 1 in]
              n409 = Equal?(x=w754, y=w753) -> (x = y?=w749:bool)
              n410 = Select(t=w748, s=w749, f=Server_Comms."Do Not Link To Server" ("Server Comms")) -> (s? t:f=w747:u32)
              n411 = local write "Server Comms"(w747) -> ()
              n412 = global write "Preference_global.vi" "Server Comms"(w747) -> ()
            }
            frame "Temperature" {
              n413 = call-poly <vilib>:"Read Key.vi"("section"=w758, "key"=w760, "refnum"=w761) -> ("value"=w759:string)  [unwired: 5 in, 3 out]
              n414 = global write "Preference_global.vi" "Temperature"(w759) -> ()
              n415 = local write "Temperature"(w759) -> ()
            }
            frame "Abs Press (mbar)" {
              n416 = call-poly <vilib>:"Read Key.vi"("section"=w762, "key"=w764, "refnum"=w765) -> ("value"=w763:string)  [unwired: 5 in, 3 out]
              n417 = global write "Preference_global.vi" "Abs Press (mbar)"(w763) -> ()
              n418 = local write "Abs Press (mbar)"(w763) -> ()
            }
            frame "EnFlo_Data_Central_Repository" {
              n419 = call-poly <vilib>:"Read Key.vi"("section"=w766, "key"=w768, "refnum"=w769) -> ("value"=w767:path)  [unwired: 5 in, 3 out]
              n420 = global write "Constants_global.vi" "EnFlo_Data_Central_Repository"(w767) -> ()
            }
            frame "Current Overhead Factor" {
              n421 = call-poly <vilib>:"Read Key.vi"("section"=w770, "key"=w772, "refnum"=w773) -> ("value"=w771:dbl)  [unwired: 5 in, 3 out]
              n422 = call "Overhead_Factor.vi"("Current Overhead Factor In"=w771, "Mode"=Overhead."Initialise totals to 3hr") -> ()  [unwired: 2 in, 1 out]
            }
            frame "Auto Calib Error fr Previous" {
              n423 = call-poly <vilib>:"Read Key.vi"("section"=w775, "key"=w777, "refnum"=w778) -> ("value"=w776:dbl)  [unwired: 5 in, 3 out]
              n424 = global write "Preference_global.vi" "% Error From Previous Calib"(w776) -> ()
              n425 = local write "% Error From Previous Calib"(w776) -> ()
            }
            frame "HaveIMAQlib" {
              n426 = call-poly <vilib>:"Read Key.vi"("section"=w780, "key"=w781, "refnum"=w782) -> ("value"=w779:bool)  [unwired: 5 in, 3 out]
              n427 = global write "Preference_global.vi" "HaveIMAQlibrary"(w779) -> ()
              n428 = local write "IMAQ?"(w779) -> ()
            }
            frame "MaxEmailsPerDay" {
              n429 = call-poly <vilib>:"Read Key.vi"("section"=w785, "default value"=u32 20, "key"=w786, "refnum"=w787) -> ("value"=w784:u32)  [unwired: 4 in, 3 out]
              n430 = local write "MaxDailyEmails"(w784) -> ()
              n431 = global write "Preference_global.vi" "MaxDailyEmails"(w784) -> ()
            }
          }
        }
        n432 = local read "Post Processing Machine"() -> (w691:bool)
        n433 = Select(t="Check file permission status", s=w691, f="is traverse setup blank?") -> (s? t:f=w689:string)
      }
      frame "is traverse setup blank?" {
        n434 = local read "Data Folder"() -> (w795:path)
        n435 = Build Path(base path=w795, name or relative path="Preferences") -> (appended path=w794:path)
        n436 = global read "Trav_pos_global.vi" "Default Traverse Setup"() -> (w789:string)
        n437 = Build Path(base path=w794, name or relative path=w797) -> (appended path=w793:path)
        n438 = List Folder(path=w793) -> (folder names=w791:string[])  [unwired: 1 in, 5 out]
        n439 = Search 1D Array(1D array=w791, element=w789) -> (index of element=w792:i32)  [unwired: 1 out]
        n440 = case shown="0, Default" w792 {
          tunnel: w791 -> [_ w803]
          tunnel: [w801 w802] -> w790
          tunnel: w789 -> [w801 _]
          frame 0, Default {
          }
          frame -1 {
            n441 = Index Array(array=w803, index=0) -> (element=w802:string)
          }
        }
        n442 = global write "Trav_pos_global.vi" "Default Traverse Setup"(w790) -> ()
      }
      frame "Please Enter new  Traverse Setup" {
        n443 = global read "Trav_pos_global.vi" "Default Traverse Setup"() -> (w807:string)
        n444 = String Length(string=w807) -> (length=w812:i32)
        n445 = In Range and Coerce(upper limit=w809, x=w812, lower limit=w810) -> (In Range?=w808:bool)  [unwired: 1 out]
        n446 = case shown="False" w808 {
          tunnel: w807 -> [w823 w831]
          tunnel: ["Please Enter new  Traverse Setup" "Update Traverse setup menu ring"] -> w811
          tunnel: [w816 w831] -> w806
          tunnel: w810 -> [w820 _]
          tunnel: w809 -> [w819 _]
          frame False {
            n447 = Format Into String(format string="Please Enter a Traverse Setup Name\nIt must be between %d and %d Characters" ("Message to user"), w820, w819) -> (resulting string=w818:string)  [unwired: 2 in, 1 out]
            n448 = call "Input_String_Dialog.vi"("Value"=w823, "Message to user"=w818) -> ("Ok Out"=w815:bool, "Output string"=w817:string)
            n449 = case shown="False" w815 {
              tunnel: w817 -> [_ w828]
              tunnel: [w824 w827] -> w816
              frame False {
                n450 = property on="Default Traverse Name" class="Ring (strict)"() -> ("Strings []"=w825:string[])  [unwired: 2 in, 2 out]
                n451 = Index Array(array=w825, index=0) -> (element=w824:string)
              }
              frame True {
                n452 = call "Fast_string_Replace.vi"("Replace match with:"="_", "Input String"=w828, "matchThis"=" " ("regular expression")) -> ("Output String"=w827:string)  [unwired: 1 in, 1 out]
              }
            }
          }
          frame True {
          }
        }
        n453 = global write "Trav_pos_global.vi" "Default Traverse Setup"(w806) -> ()
      }
      frame "Update Traverse setup menu ring" {
        n454 = local read "Data Folder"() -> (w843:path)
        n455 = Build Path(base path=w843, name or relative path="Preferences") -> (appended path=w842:path)
        n456 = Build Path(base path=w842, name or relative path=w837) -> (appended path=w836:path)
        n457 = global read "Trav_pos_global.vi" "Default Traverse Setup"() -> (w839:string)
        n458 = call "Get Traverse Names.vi"("Traverse name"="", "Traverse\nSetup\nFolder"=w836) -> ("Traverse Names"=w835:string[])  [unwired: 1 out]
        n459 = Build Array (concatenate)(w835, "--New Traverse Setup--") -> (w840:string[])
        n460 = Search 1D Array(1D array=w840, element=w839) -> (index of element=w845:i32)  [unwired: 1 out]
        n461 = case shown="-1" w845 {
          selector: w845 -> [w850 _]
          tunnel: [w850 0] -> w847
          tunnel: w840 -> [w851 w854]
          tunnel: w839 -> [_ w853]
          tunnel: [w851 w852] -> w838
          frame 0, Default {
          }
          frame -1 {
            n462 = Build Array (concatenate)(w853, w854) -> (w852:string[])
          }
        }
        n463 = local write "Default Traverse Name"(w847) -> ()
        n464 = property on="Default Traverse Name" class="Ring (strict)"("Strings []"=w838) -> ()  [unwired: 2 in, 2 out]
      }
      frame "Create Traverse setup" {
        n465 = local read "Templates"() -> (w857:path)
        n466 = Build Path(base path=w857, name or relative path="All_Traverses") -> (appended path=w859:path)
        n467 = stacked-sequence {
          seq-local: [w865 _] -> [_ w890]
          seq-local: [w864 _] -> [_ _]
          tunnel: w859 -> [w867 _]
          tunnel: w857 -> [_ w889]
          frame #0 {
            w872 = "Default_Space_file.xls" ("name or relative path")
            w863 = "Traverse_Setup.xls" ("name or relative path")
            n468 = global read "Trav_pos_global.vi" "Default Traverse Setup"() -> (w864:string)
            n469 = global read "Constants_global.vi" "Traverse folder"() -> (w876:path)
            n470 = Build Path(base path=w876, name or relative path=w864) -> (appended path=w865:path)
            n471 = Build Path(base path=w865, name or relative path="Trav_Space_Files") -> (appended path=w873:path)
            n472 = Build Path(base path=w867, name or relative path=w863) -> (appended path=w866:path)
            n473 = Build Path(base path=w867, name or relative path=w872) -> (appended path=w870:path)
            n474 = Build Path(base path=w873, name or relative path=w872) -> (appended path=w869:path)
            n475 = Build Path(base path=w865, name or relative path=w863) -> (appended path=w868:path)
            n476 = call "Does_file_exist_(simple).vi"("Pathname"=w869) -> ("exists?"=w871:bool)
            n477 = case shown="False" w871 {
              tunnel: w870 -> [w879 _]
              tunnel: w869 -> [w878 _]
              frame False {
                n478 = call "Create_directory_path.vi"("Path name"=w878) -> ("Path name Out"=w877:path)  [unwired: 2 in, 1 out]
                n479 = Copy(10:w877, 11:w879) -> ()  [unwired: 1 in, 5 out]
              }
              frame True {
              }
            }
            n480 = call "Does_file_exist_(simple).vi"("Pathname"=w868) -> ("exists?"=w875:bool)
            n481 = case shown="False" w875 {
              tunnel: w866 -> [w886 _]
              tunnel: w868 -> [w882 _]
              tunnel: w864 -> [w885 _]
              frame False {
                n482 = call "Create_directory_path.vi"("Path name"=w882) -> ("Path name Out"=w881:path)  [unwired: 2 in, 1 out]
                n483 = call "Read_File_Simple.vi"("Filename"=w886) -> ("string"=w884:string)  [unwired: 2 in, 7 out]
                n484 = call "Fast_string_Replace.vi"("Replace match with:"=w885, "Input String"=w884, "matchThis"="A_Tunnel" ("regular expression")) -> ("Output String"=w880:string)  [unwired: 1 in, 1 out]
                n485 = call "Write Characters with check.vi"("String to Write"=w880, "file (use dialog)"=w881) -> ()  [unwired: 2 in, 1 out]
              }
              frame True {
              }
            }
          }
          frame #1 {
            w888 = "Traverse_Preferences.txt" ("name or relative path")
            n486 = Build Path(base path=w890, name or relative path=w888) -> (appended path=w887:path)
            n487 = Build Path(base path=w889, name or relative path=w888) -> (appended path=w891:path)
            n488 = call "Does_file_exist_(simple).vi"("Pathname"=w887) -> ("exists?"=w892:bool)
            n489 = case shown="False" w892 {
              tunnel: w891 -> [w895 _]
              tunnel: w887 -> [w894 _]
              frame False {
                n490 = call "Create_directory_path.vi"("Path name"=w894) -> ("Path name Out"=w893:path)  [unwired: 2 in, 1 out]
                n491 = Copy(10:w893, 11:w895) -> ()  [unwired: 1 in, 5 out]
              }
              frame True {
              }
            }
          }
        }
      }
      frame "Check file permission status" {
        # "Does not do this now  Dec 2021 PH"
        n492 = local read "Post Processing Machine"() -> (w897:bool)
        n493 = case shown="\"Save Preferences to file\", Default" w898 {
          tunnel: [w903 w907] -> w899
          tunnel: w897 -> [w902 w906]
          frame "Save Preferences to file", Default {
            n494 = Select(t="Save Preference File", s=w902, f="CreateAndTestFolders") -> (s? t:f=w903:string)
          }
          frame "Load, Edit then Save" {
            n495 = Select(t="Data Folder Changed?", s=w906, f="What next1") -> (s? t:f=w907:string)
          }
        }
      }
      frame "What next1" {
        n496 = property on="Rig Setup" class="Ring (strict)"() -> ("Strings []"=w912:string[])  [unwired: 2 in, 2 out]
        n497 = Array Size(array=w912) -> (size(s)=w916:i32)
        n498 = Decrement(x=w916) -> (x-1=w915:i32)
        n499 = Equal?(x=w915, y="Rig Setup") -> (x = y?=w914:bool)
        n500 = case shown="False" w914 {
          tunnel: [w920 "Please Enter New Rig Name" ("t")] -> w913
          tunnel: w912 -> [w923 _]
          tunnel: "Rig Setup" -> [w922 _]
          frame False {
            n501 = global read "Preference_global.vi" "Rig Setup"() -> (w924:string)
            n502 = Index Array(array=w923, index=w922) -> (element=w919:string)
            n503 = Not Equal?(x=w919, y=w924) -> (x != y?=w921:bool)
            n504 = case shown="False" w921 {
              tunnel: ["What next2" ("f") "Update Rig setup menu ring" ("t")] -> w920
              tunnel: w919 -> [_ w926]
              frame False {
              }
              frame True {
                n505 = global write "Preference_global.vi" "Rig Setup"(w926) -> ()
              }
            }
          }
          frame True {
            n506 = global write "Preference_global.vi" "Rig Setup"("") -> ()
          }
        }
      }
      frame "What next2" {
        n507 = property on="Default Traverse Name" class="Ring (strict)"() -> ("Strings []"=w932:string[])  [unwired: 2 in, 2 out]
        n508 = Array Size(array=w932) -> (size(s)=w936:i32)
        n509 = Decrement(x=w936) -> (x-1=w935:i32)
        n510 = Equal?(x=w935, y="Default Traverse Name") -> (x = y?=w934:bool)
        n511 = case shown="False" w934 {
          tunnel: [w940 "Please Enter new  Traverse Setup" ("t")] -> w933
          tunnel: w932 -> [w944 _]
          tunnel: "Default Traverse Name" -> [w943 _]
          frame False {
            n512 = global read "Trav_pos_global.vi" "Default Traverse Setup"() -> (w942:string)
            n513 = Index Array(array=w944, index=w943) -> (element=w939:string)
            n514 = Not Equal?(x=w939, y=w942) -> (x != y?=w941:bool)
            n515 = case shown="False" w941 {
              tunnel: [w945 "Update Traverse setup menu ring" ("t")] -> w940
              tunnel: w939 -> [_ w949]
              frame False {
                n516 = Select(t="Select User Name", s="Change?", f="Data Folder Changed?") -> (s? t:f=w945:string)
              }
              frame True {
                n517 = global write "Trav_pos_global.vi" "Default Traverse Setup"(w949) -> ()
              }
            }
          }
          frame True {
            n518 = global write "Trav_pos_global.vi" "Default Traverse Setup"("") -> ()
          }
        }
      }
      frame "Data Folder Changed?" {
        w956 = "Please Select your data folder"
        n519 = while {
          shift-right: [w971] -> _
          shift-left: _ -> [w970]
          tunnel: [w969] -> w958
          stop <- TRUE stop-if-true
          n520 = local read "Post Processing Machine"() -> (w971:bool)
          n521 = Not Equal?(x=w971, y=w970) -> (x != y?=w969:bool)
        }
        n522 = global read "Constants_global.vi" "Data Folder"() -> (w961:path)
        n523 = local read "Data Folder"() -> (w962:path)
        n524 = Not Equal?(x=w961, y=w962) -> (x != y?=w954:bool)
        n525 = Select(t=w956, s=w954, f="Has OK has been pressed?") -> (s? t:f=w955:string)
        n526 = case shown="False" w958 {
          tunnel: [w965 w967] -> w957
          tunnel: w956 -> [_ w967]
          tunnel: w955 -> [w965 _]
          frame False {
          }
          frame True {
            n527 = global write "Preference_global.vi" "Rig Setup"("") -> ()
          }
        }
        n528 = property on="OK" class="Bool (strict)"("Visible"=TRUE) -> ()  [unwired: 2 in, 2 out]
      }
      frame "Has OK has been pressed?" {
        n529 = stacked-sequence {
          tunnel: [_ "OK" _ _] -> w974
          frame #0 {
            n530 = Wait (ms)(milliseconds to wait=u32 100) -> ()  [unwired: 1 out]
          }
          frame #1 {
          }
          frame #2 {
            n531 = property on="Select Local Cameras to Log" class="LstBox (strict)"() -> ("Item Names"=w982:string[])  [unwired: 2 in, 2 out]
            n532 = for {
              tunnel: "Select Local Cameras to Log" -> [w985] mode=indexing
              tunnel: w982 -> [w984]
              tunnel: [w983] -> w980 mode=indexing
              n533 = Index Array(array=w984, index=w985) -> (element=w983:string)
            }
            n534 = global write "CamServer global.vi" "Demanded Local cameras"(w980) -> ()
          }
          frame #3 {
            n535 = case shown="True" "View Local Cameras Now" {
              frame False {
              }
              frame True {
                n536 = local write "View Local Cameras Now"(FALSE ("View Local Cameras Now")) -> ()
                n537 = call "Save Local Images.vi"("Save Images"=FALSE) -> ()  [unwired: 2 in, 2 out]
              }
            }
          }
        }
        n538 = local read "Post Processing Machine"() -> (w975:bool)
        n539 = case shown="True" w974 {
          tunnel: w975 -> [w990 w996]
          tunnel: [w989 w993] -> w973
          frame False {
            n540 = Select(t="Data Folder Changed?", s=w990, f="What next1") -> (s? t:f=w989:string)
          }
          frame True {
            n541 = Select(t="Save Preference File", s=w996, f="CreateAndTestFolders") -> (s? t:f=w993:string)
          }
        }
      }
      frame "CreateAndTestFolders" {
        n542 = global read "Preference_global.vi" "Site Specific String (Blank if Surrey)"() -> (w997:string)
        n543 = case shown="\"CPP\"" w997 {
          frame "CPP" {
            # "We'll create project folders as soon as we know we're actually going to use them..."
          }
          frame "Surrey", Default {
            n544 = for {
              tunnel: cluster{"String":string, "String":string}[] [{"String"="Raw_Cal", "String"="Raw_Calibrations"}, {"String"="Raw_Meas", "String"="Raw_Measurements"}, {"String"="Res", "String"="Results"}, {"String"="Cal", "String"="Calibrations"}, {"String"="Cmd", "String"="Commands"}, {"String"="Pic", "String"="Pictures"}, {"String"="Video", "String"="Videos"}, {"String"="Doc", "String"="Documents"}, {"String"="PP", "String"="Results_Post_Processed"}] ("array of clusters") -> [w1005] mode=indexing
              n545 = Unbundle(w1005) -> ("String"=w1004:string, "String"=w1003:string)
              n546 = call "Data_folder_Path.vi"("Data Type"=w1003, "Short_Name"=w1004) -> ("Data Folder"=w1006:path)  [unwired: 4 in]
              n547 = Build Path(base path=w1006, name or relative path="Test" ("Substring")) -> (appended path=w1008:path)
              n548 = call "Create_directory_path.vi"("Path name"=w1008) -> ()  [unwired: 2 in, 2 out]
            }
          }
        }
      }
      frame "Save Preference File" {
        n549 = for {
          tunnel: w1015 -> [w1028] mode=indexing
          tunnel: w1010 -> [w1027]
          tunnel: w1009 -> [w1026]
          n550 = case shown="\"Local Cameras to Log\"" w1028 {
            selector: w1028 -> [w1029 w1032 w1038 w1042 w1044 w1048 w1052 w1056 w1060 w1065 w1069 w1073 w1080 w1087 w1093 w1098 w1102 w1106 w1110]
            tunnel: w1026 -> [_ w1033 w1036 w1039 w1046 w1050 w1053 w1058 w1062 w1067 w1070 w1074 w1082 w1089 w1090 w1095 w1100 w1105 w1109]
            tunnel: w1027 -> [_ w1031 w1037 w1040 w1045 w1049 w1054 w1057 w1061 w1066 w1071 w1075 w1081 w1088 w1091 w1096 w1099 w1104 w1108]
            frame "No Match", Default {
              n551 = call "Was_string_matched.vi"("Match Error"=TRUE, "Variable name"=w1029) -> ()  [unwired: 1 in]
            }
            frame "Server address" {
              n552 = global write "Preference_global.vi" "Server address"("Server address") -> ()
              n553 = call-poly <vilib>:"Write Key.vi"("section"=w1033, "value"="Server address", "key"=w1032, "refnum"=w1031) -> ()  [unwired: 5 in, 3 out]
            }
            frame "Server port number" {
              n554 = global write "Preference_global.vi" "Server port number"("Server port number") -> ()
              n555 = call-poly <vilib>:"Write Key.vi"("section"=w1036, "value"="Server port number", "key"=w1038, "refnum"=w1037) -> ()  [unwired: 5 in, 3 out]
            }
            frame "Default Source Establishment Time (s)" {
              n556 = global write "Preference_global.vi" "Default Source Establishment Time (s)"("Default Source Establishment Time (s)") -> ()
              n557 = call-poly <vilib>:"Write Key.vi"("section"=w1039, "value"="Default Source Establishment Time (s)", "key"=w1042, "refnum"=w1040) -> ()  [unwired: 5 in, 3 out]
            }
            frame "Tunnel Speed Control" {
              n558 = global write "Preference_global.vi" "Tunnel Speed Control"("Tunnel Speed Control") -> ()
              n559 = call-poly <vilib>:"Write Key.vi"("section"=w1046, "value"="Tunnel Speed Control", "key"=w1044, "refnum"=w1045) -> ()  [unwired: 5 in, 3 out]
            }
            frame "Traverse to Traverse Collision Detection" {
              n560 = global write "Preference_global.vi" "Traverse to Traverse Collision Detection"("Traverse to Traverse Collision Detection") -> ()
              n561 = call-poly <vilib>:"Write Key.vi"("section"=w1050, "value"="Traverse to Traverse Collision Detection", "key"=w1048, "refnum"=w1049) -> ()  [unwired: 5 in, 3 out]
            }
            frame "Log Cameras if available" {
              n562 = global write "Preference_global.vi" "Log Cameras if available"("Log Cameras if available") -> ()
              n563 = call-poly <vilib>:"Write Key.vi"("section"=w1053, "value"="Log Cameras if available", "key"=w1052, "refnum"=w1054) -> ()  [unwired: 5 in, 3 out]
            }
            frame "Use Triangle and Tree Collision Code" {
              n564 = global write "Preference_global.vi" "Use New Collision Code"("Use New Collision Code") -> ()
              n565 = call-poly <vilib>:"Write Key.vi"("section"=w1058, "value"="Use New Collision Code", "key"=w1056, "refnum"=w1057) -> ()  [unwired: 5 in, 3 out]
            }
            frame "Local Cameras to Log" {
              n566 = global read "CamServer global.vi" "Demanded Local cameras"() -> (w1063:T15[])
              n567 = call "Put_Array_into_String.vi"("String array"=w1063) -> ("String Value"=w1059:string)
              n568 = call-poly <vilib>:"Write Key.vi"("section"=w1062, "value"=w1059, "key"=w1060, "refnum"=w1061) -> ()  [unwired: 5 in, 3 out]
            }
            frame "SMTP server IP address" {
              n569 = global write "Preference_global.vi" "SMTP server IP address"("SMTP server IP address") -> ()
              n570 = call-poly <vilib>:"Write Key.vi"("section"=w1067, "value"="SMTP server IP address", "key"=w1065, "refnum"=w1066) -> ()  [unwired: 5 in, 3 out]
            }
            frame "Default Traverse Name" {
              n571 = global read "Trav_pos_global.vi" "Default Traverse Setup"() -> (w1068:string)
              n572 = call-poly <vilib>:"Write Key.vi"("section"=w1070, "value"=w1068, "key"=w1069, "refnum"=w1071) -> ()  [unwired: 5 in, 3 out]
            }
            frame "Server Comms" {
              n573 = global write "Preference_global.vi" "Server Comms"("Server Comms") -> ()
              n574 = call-poly <vilib>:"Write Key.vi"("section"=w1074, "value"="Server Comms", "key"=w1073, "refnum"=w1075) -> ()  [unwired: 5 in, 3 out]
            }
            frame "Temperature" {
              n575 = Empty String/Path?(string/path="Temperature") -> (empty?=w1079:bool)
              n576 = Select(t="manual:Temp:C", s=w1079, f="Temperature") -> (s? t:f=w1077:string)
              n577 = global write "Preference_global.vi" "Temperature"(w1077) -> ()
              n578 = call-poly <vilib>:"Write Key.vi"("section"=w1082, "value"=w1077, "key"=w1080, "refnum"=w1081) -> ()  [unwired: 5 in, 3 out]
            }
            frame "Abs Press (mbar)" {
              n579 = Empty String/Path?(string/path="Abs Press (mbar)") -> (empty?=w1085:bool)
              n580 = Select(t="manual:Press:mBar", s=w1085, f="Abs Press (mbar)") -> (s? t:f=w1086:string)
              n581 = global write "Preference_global.vi" "Abs Press (mbar)"(w1086) -> ()
              n582 = call-poly <vilib>:"Write Key.vi"("section"=w1089, "value"=w1086, "key"=w1087, "refnum"=w1088) -> ()  [unwired: 5 in, 3 out]
            }
            frame "Current Overhead Factor" {
              n583 = call "Overhead_Factor.vi"("Mode"=Overhead."Read Current Overhead") -> ("Current Overhead Factor"=w1092:dbl)  [unwired: 3 in]
              n584 = call-poly <vilib>:"Write Key.vi"("section"=w1090, "value"=w1092, "key"=w1093, "refnum"=w1091) -> ()  [unwired: 5 in, 3 out]
            }
            frame "Auto Calib Error fr Previous" {
              n585 = global write "Preference_global.vi" "% Error From Previous Calib"("% Error From Previous Calib") -> ()
              n586 = call-poly <vilib>:"Write Key.vi"("section"=w1095, "value"="% Error From Previous Calib", "key"=w1098, "refnum"=w1096) -> ()  [unwired: 5 in, 3 out]
            }
            frame "EnFlo_Data_Central_Repository" {
              n587 = global read "Constants_global.vi" "EnFlo_Data_Central_Repository"() -> (w1101:path)
              n588 = call-poly <vilib>:"Write Key.vi"("section"=w1100, "value"=w1101, "key"=w1102, "refnum"=w1099) -> ()  [unwired: 5 in, 3 out]
            }
            frame "HaveIMAQlib" {
              n589 = call-poly <vilib>:"Write Key.vi"("section"=w1105, "value"="IMAQ?", "key"=w1106, "refnum"=w1104) -> ()  [unwired: 5 in, 3 out]
            }
            frame "MaxEmailsPerDay" {
              n590 = global write "Preference_global.vi" "MaxDailyEmails"("MaxDailyEmails") -> ()
              n591 = call-poly <vilib>:"Write Key.vi"("section"=w1109, "value"="MaxDailyEmails", "key"=w1110, "refnum"=w1108) -> ()  [unwired: 5 in, 3 out]
            }
          }
        }
        n592 = case shown="\"Load, Edit then Save\"" w1013 {
          tunnel: [TRUE TRUE TRUE] -> w1012
          frame "Load, Edit then Save" {
            n593 = Current VI's Path() -> (path=w1022:path)
            n594 = call "Open_Close_Front_Panel.ph.vi"("openWindow (T)"=FALSE ("Front Panel Window:Open"), "VI path"=w1022) -> ()  [unwired: 1 in, 1 out]
          }
          frame "Load Preferences from file" {
          }
          frame "Save Preferences to file" {
          }
        }
        n595 = call "Date_and_Time_to_string.vi"() -> ("dateTime"=w1011:T16)  [unwired: 4 in, 1 out]
        n596 = for {
          tunnel: w1011 -> [w1020] mode=indexing
          tunnel: w1010 -> [w1017]
          tunnel: w1009 -> [w1016]
          n597 = Unbundle(w1020) -> ("Label.Text"=w1019:string, "date/time string"=w1018:string)
          n598 = call-poly <vilib>:"Write Key.vi"("section"=w1016, "value"=w1018, "key"=w1019, "refnum"=w1017) -> ()  [unwired: 5 in, 3 out]
        }
      }
      frame "Save SW Preferences" {
        w1113 = "Bootstrap"
        n599 = local read "EnFlo SW Preferences"() -> (w1119:path)
        n600 = call <vilib>:"Open Config Data.vi"("configuration file path"=w1119) -> ("refnum"=w1130:T12)  [unwired: 8 in, 2 out]
        n601 = call "Date_and_Time_to_string.vi"() -> ("dateTime"=w1131:T16)  [unwired: 4 in, 1 out]
        n602 = for {
          tunnel: w1131 -> [w1143] mode=indexing
          tunnel: "Timestamp" -> [w1140]
          tunnel: w1130 -> [w1139]
          tunnel: [w1138] -> w1129
          n603 = Unbundle(w1143) -> ("Label.Text"=w1142:string, "date/time string"=w1141:string)
          n604 = call-poly <vilib>:"Write Key.vi"("section"=w1140, "value"=w1141, "key"=w1142, "refnum"=w1139) -> ("refnum out"=w1138:T12)  [unwired: 5 in, 2 out]
        }
        n605 = local read "Post Processing Machine"() -> (w1123:bool)
        n606 = call-poly <vilib>:"Write Key.vi"("section"=w1113, "value"="Data Folder", "key"=w1126, "refnum"=w1129) -> ("refnum out"=w1128:T12)  [unwired: 5 in, 2 out]
        n607 = global read "Preference_global.vi" "Rig Setup"() -> (w1117:string)
        n608 = call-poly <vilib>:"Write Key.vi"("section"=w1113, "value"=w1117, "key"=w1116, "refnum"=w1128) -> ("refnum out"=w1118:T12)  [unwired: 5 in, 2 out]
        n609 = global read "Preference_global.vi" "User_Name"() -> (w1121:string)
        n610 = global read "Preference_global.vi" "Server Comms"() -> (w1135:T2)
        n611 = call-poly <vilib>:"Write Key.vi"("section"=w1113, "value"=w1123, "key"=w1124, "refnum"=w1118) -> ("refnum out"=w1127:T12)  [unwired: 5 in, 2 out]
        n612 = call-poly <vilib>:"Write Key.vi"("section"=w1113, "value"=w1121, "key"=w1122, "refnum"=w1127) -> ("refnum out"=w1115:T12)  [unwired: 5 in, 2 out]
        n613 = case shown="\"Server Link Healthy\"" w1135 {
          tunnel: ["Update Served VI file" "Update Local Adam Table"] -> w1134
          frame "Server Link Healthy" {
          }
          frame "Do Not Link To Server" {
          }
        }
        n614 = call-poly <vilib>:"Write Key.vi"("section"=w1113, "value"="FixedUserName", "key"=w1112, "refnum"=w1115) -> ("refnum out"=w1114:T12)  [unwired: 5 in, 2 out]
        n615 = call <vilib>:"Close Config Data.vi"("refnum"=w1114) -> ()  [unwired: 9 in, 2 out]
        n616 = case shown="True" "Reset Email Counter" {
          tunnel: "Reset Email Counter" -> [_ w1144]
          frame False {
          }
          frame True {
            n617 = global write "Preference_global.vi" "Unblock Email"(w1144) -> ()
          }
        }
      }
      frame "Update Local Adam Table" {
        n618 = stacked-sequence {
          seq-local: [w1156 _] -> [_ w1172]
          tunnel: ["Update Served VI file" _] -> w1148
          frame #0 {
            w1156 = T17 {"Ch Name"="", "Type"="", "Function"=enum."Analogue Input", "Ch State"=enum."On", "Calibration type"="", "A"=0.0, "B"=0.0, "C"=0.0, "D"=0.0, "Comments"="", "Address"={"Main"=0, "Ch."=0, "Sub"=0, "Port Name"=""}, "String"="", "Duty"=0} ("Ch Discription")
            n619 = global read "Preference_global.vi" "Abs Press (mbar)"() -> (w1153:string)
            n620 = global read "Preference_global.vi" "Temperature"() -> (w1154:string)
            n621 = Bundle By Name(cluster=w1156, "Type"=T9 "", "Calibration type"=T8 "", "A"=1.0) -> (w1157:T17)
            n622 = Build Array(w1154, w1153) -> (w1152:string[])
            n623 = for {
              tunnel: [w1163] -> w1155 mode=indexing
              tunnel: w1157 -> [w1162]
              tunnel: w1152 -> [w1161] mode=indexing
              n624 = Bundle By Name(cluster=w1162, "Ch Name"=w1161) -> (w1163:T17)
            }
            n625 = call "Update_Ch_Discription_client.vi"("Channels to update In"=w1155) -> ()  [unwired: 1 out]
          }
          frame #1 {
            n626 = global read "Preference_global.vi" "Rig Setup"() -> (w1167:string)
            n627 = call "Get_Current_Scan_client.vi"() -> ("Ch Description Array"=w1173:T17[])  [unwired: 2 in, 3 out]
            n628 = Match Pattern(string=w1167, regular expression="-") -> (before substring=w1166:string)  [unwired: 4 out]
            n629 = Format Into String(format string="%s Metadata:" ("Format String"), w1166) -> (resulting string=w1164:string)  [unwired: 2 in, 1 out]
            n630 = Initialize Array(w1172, 0 ("dimension size")) -> (w1170:T17[])
            n631 = for {
              shift-right: [w1184] -> w1169
              shift-left: w1170 -> [w1185]
              tunnel: w1173 -> [w1176] mode=indexing
              tunnel: w1164 -> [w1183]
              tunnel: "Metadata:" ("Format String") -> [w1182]
              n632 = Unbundle By Name(w1176) -> ("Ch Name"=w1175:string)
              n633 = Match Pattern(string=w1175, regular expression=w1183) -> (offset past match=w1180:i32)  [unwired: 4 out]
              n634 = Match Pattern(string=w1175, regular expression=w1182) -> (offset past match=w1181:i32)  [unwired: 4 out]
              n635 = Greater Or Equal To 0?(x=w1181) -> (x >= 0?=w1178:bool)
              n636 = Less Than 0?(x=w1180) -> (x < 0?=w1179:bool)
              n637 = And(x=w1179, y=w1178) -> (x .and. y?=w1177:bool)
              n638 = case shown="True" w1177 {
                tunnel: w1185 -> [w1186 w1191]
                tunnel: [w1186 w1190] -> w1184
                tunnel: w1176 -> [_ w1189]
                frame False {
                }
                frame True {
                  n639 = Bundle By Name(cluster=w1189, "Ch State"=Channel_State."Off") -> (w1187:T17)
                  n640 = Build Array (concatenate)(w1191, w1187) -> (w1190:T17[])
                }
              }
            }
            n641 = call "Update_Ch_Discription_client.vi"("Channels to update In"=w1169) -> ()  [unwired: 1 out]
          }
        }
      }
      frame "Update Served VI file" {
        n642 = global read "Preference_global.vi" "Rig Setup"() -> (w1193:string)
        n643 = case shown="\"Zephyr\"" w1193 {
          tunnel: [GMU_Gas_Line_Name."GMU2 Source" ("Gas Line Name") GMU_Gas_Line_Name."GMU1 Source" ("Gas Line Name") GMU_Gas_Line_Name."CPP GRC-A" ("Gas Line Name") GMU_Gas_Line_Name."CPP GRC-B" ("Gas Line Name") GMU_Gas_Line_Name."CPP GRC-B" ("Gas Line Name")] -> w1192
          frame Default {
          }
          frame "EnFlo_Tunnel" {
          }
          frame "GDE" {
          }
          frame "GDW" {
          }
          frame "Zephyr" {
          }
        }
        "Default Gas Line Name" <- w1192
        n644 = call "Setup_Filepath.vi"("Setup File Type"=Setup_Filetype."General", "Filename in"=w1196) -> ("Filename Out"=w1195:path)  [unwired: 1 out]
        n645 = global write "Trav_pos_global.vi" "Default Gas Line Name"(w1192) -> ()
        n646 = Build Array("Served:VI:Name", "Served:VI:Path", "Server:IP Number:& Port No") -> (w1200:string[])
        n647 = stacked-sequence {
          seq-local: [w1210 _ _ _] -> [_ _ w1220 _]
          seq-local: [_ w1217 _ _] -> [_ _ w1221 _]
          seq-local: [_ _ w1222 _] -> [_ _ _ w1246]
          tunnel: w1200 -> [w1212 w1218 _ w1247]
          tunnel: w1195 -> [w1211 _ _ w1248]
          tunnel: w1196 -> [_ w1214 _ _]
          frame #0 {
            n648 = call "Read_Ch_data_file.vi"("Present Channels"=w1212, "Output"=enum16{"All Ch data", "The last few rows"}."All Ch data", "Filename"=w1211) -> ("Channel Values"=w1210:string[][])  [unwired: 2 in, 4 out]
          }
          frame #1 {
            n649 = local read "Templates"() -> (w1216:path)
            n650 = Build Path(base path=w1216, name or relative path=w1214) -> (appended path=w1215:path)
            n651 = call "Read_Ch_data_file.vi"("Present Channels"=w1218, "Output"=enum16{"All Ch data", "The last few rows"}."All Ch data", "Filename"=w1215) -> ("Channel Values"=w1217:string[][])  [unwired: 2 in, 4 out]
          }
          frame #2 {
            n652 = Index Array(array=w1220, index (col)=0 ("Index")) -> (element=w1225:string[])  [unwired: 1 in]
            n653 = To Upper Case(1:w1221) -> (0:w1223:string[][])
            n654 = To Upper Case(1:w1225) -> (0:w1224:string[])
            n655 = for {
              tunnel: w1224 -> [w1228]
              tunnel: w1221 -> [w1233] mode=indexing
              tunnel: w1223 -> [w1227] mode=indexing
              tunnel: [w1230] -> w1222 mode=indexing
              tunnel: w1220 -> [w1229]
              n656 = Index Array(array=w1227, index=0 ("Index")) -> (element=w1231:string)
              n657 = Search 1D Array(1D array=w1228, element=w1231) -> (index of element=w1232:i32)  [unwired: 1 out]
              n658 = case shown="0, Default" w1232 {
                tunnel: w1233 -> [w1242 w1243]
                tunnel: w1232 -> [w1239 _]
                tunnel: [w1235 w1243] -> w1230
                tunnel: w1229 -> [w1240 _]
                frame 0, Default {
                  n659 = Index Array(array=w1240, index (row)=w1239, index (col)=2 ("Index")) -> (element=w1237:string)
                  n660 = Array Subset(array=w1242, length=2) -> (w1236:string[])  [unwired: 1 in]
                  n661 = Build Array (concatenate)(w1236, w1237) -> (w1235:string[])
                }
                frame -1 {
                }
              }
            }
          }
          frame #3 {
            w1244 = FALSE  # Append last row only
            w1245 = FALSE  # exists?
            n662 = call "Write_Ch_data_file.vi"("Append last row only"=w1244, "exists?"=w1245, "Channel Values"=w1246, "Channel names"=w1247, "Filename"=w1248) -> ()  [unwired: 3 in, 4 out]
          }
        }
      }
      frame "Initialise Globals" {
        w1264 = TRUE  # OK
        n663 = global read "Constants_global.vi" "ADAM setups folder"() -> (w1270:path)
        n664 = property on="ADAM Setup File" class="Ring (strict)"() -> ("Strings []"=w1265:string[])  [unwired: 2 in, 2 out]
        n665 = Build Path(base path=w1270, name or relative path="Setup_Files") -> (appended path=w1268:path)
        n666 = Build Path(base path=w1268, name or relative path="Selected_Filename.txt" ("Substring")) -> (appended path=w1252:path)
        n667 = Index Array(array=w1265, index="ADAM Setup File") -> (element=w1251:string)
        n668 = call "Get_users_email_addresses.vi"("OK"=w1264) -> ()  [unwired: 5 out]
        n669 = global read "Constants_global.vi" "All_Users"() -> (w1263:path)
        n670 = Build Path(base path=w1263, name or relative path="Current_Username") -> (appended path=w1250:path)
        n671 = global read "Preference_global.vi" "User_Name"() -> (w1249:string)
        n672 = call "Write Characters with check.vi"("String to Write"=w1251, "file (use dialog)"=w1252) -> ()  [unwired: 2 in, 1 out]
        n673 = call "Write Characters with check.vi"("String to Write"=w1249, "file (use dialog)"=w1250) -> ()  [unwired: 2 in, 1 out]
        n674 = call "Setup_Filepath.vi"("Setup File Type"=Setup_Filetype."General", "Filename in"="Current_Project.txt") -> ("Filename Out"=w1259:path)  [unwired: 1 out]
        n675 = Read from Text File(file (use dialog)=w1259) -> (text=w1257:string)  [unwired: 3 in, 3 out]
        n676 = call "Add_filename_suffix.vi"("Filename"=w1257) -> ("Base name"=w1255:string)  [unwired: 1 in, 3 out]
        n677 = Scan From String(format string="FixedProject=%s" ("regular expression"), input string=w1255, default 1=w1255) -> (output 1=w1254:string)  [unwired: 2 in, 3 out]
        n678 = global write "Preference_global.vi" "Project Name"(w1254) -> ()
        n679 = call "Served_Global.vi"("Mode"=Serveds."Load Global From File") -> ()  [unwired: 3 out]
      }
    }
    "currentCase" <- w18
  }
  n680 = stacked-sequence {
    seq-local: [w1274 _] -> [_ w1276]
    tunnel: w4 -> [w1275 _]
    frame #0 {
      n681 = call <vilib>:"Close Config Data.vi"("refnum"=w1275) -> ()  [unwired: 9 in, 2 out]
      n682 = local read "Copy of Current User Preferences"() -> (w1274:path)
      n683 = Delete(path (use dialog)=w1274) -> ()  [unwired: 4 in, 3 out]
    }
    frame #1 {
      n684 = local read "prefsPath"() -> (w1277:path)
      n685 = Copy(10:w1276, 11:w1277) -> ()  [unwired: 3 in, 3 out]
    }
  }
